vi "sub_breakdown-check.vi"(7 "breakdown type":T1=enum."input pwr", 8 "error in (no error)":errorcluster) -> (0 "error out":errorcluster)   [LabVIEW 2019]
uses:
  breakdown.ctl
  _ctrl/rw.ctl
  _ctrl/init-r-w.ctl
  SubVIs/common/_ctrl/system-status.ctl
  _ctrl/DSP_action.ctl
  _ctrl/create-rw-close.ctl
  _ctrl/start.ctl
  common/shutdown-type.ctl
  Devices/NI Board/cDAQ-9476 DO/cnt_Relay.ctl
  SubVIs/common/hw-control.ctl
  SubVIs/common/cmd_tablecnt.ctl
  SubVIs/count/cmd_count.ctl
  SubVIs/common/Glob_Ref.vi
  common/Global_params.vi
panel:
  out "부하전압":dbl
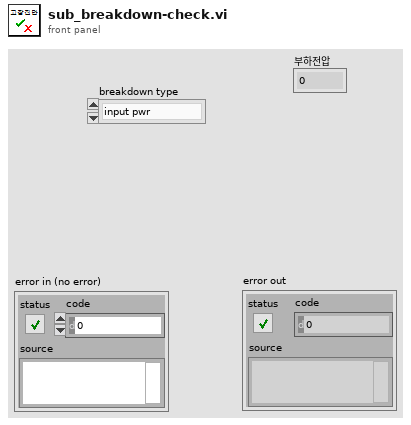
[diagram p1: front panel]
types:
  T1 = typedef "breakdown.ctl" = enum16{"DL950 items", "input pwr", "output pwr", "output pwr_adv"}
  T2 = typedef "rw.ctl" = enum16{"read", "write"}
  T3 = typedef "Breakdown-Spec.ctl" = cluster{"제어단 단선 Irms[mA](이하)":dbl, "제어단 특성 전류 Irms[mA] Max":dbl, "제어단 특성 전류 Irms[mA] Min":dbl, "출력단 단선 Irms[mA](이하)":dbl, "출력단 특성 전류 Irms[mA]  Max":dbl, "출력단 특성전류 Irms[mA]  Min":dbl, "온도[degree]":dbl}
  T4 = typedef "Testing-info.ctl" = cluster{"전체채널수":u8, "현재채널번호":u8, "Irms":dbl, "입력전압":dbl, "입력전류":dbl, "출력전압":dbl, "출력전류":dbl, "온도":dbl, "제어단 단선":bool, "제어단 단락":bool, "제어단 특성변화":bool, "출력단 단선":bool, "출력단 단락":bool, "출력단 특성변화":bool, "출력단 전압":bool, "카운트 일치":bool, "Irms 판정":bool, "온도":bool, "테스트 회수":u32, "TestType":T5, "현재회수":u32, "Ch selection":cluster{"1ch":bool, "2ch":bool, "3ch":bool, "4ch":bool, "5ch":bool, "6ch":bool}, "반복":u32, "Path":path, "파일생성주기":u32, "start time":dbl, "stop time":dbl, "현재반복회수":u32, "NG":cluster{"입출력 카운트":bool, "출력전류RMS":bool}}
  T5 = typedef "sequence_single.ctl" = enum16{"Register", "RC", "B1", "B2", "B3", "Oper_LV", "Oper_HV", "ContR_LV"}
  T6 = typedef "init-r-w.ctl" = enum16{"init", "read", "write"}
  T7 = typedef "DSP_action.ctl" = enum16{"False", "cont", "on", "off", "discont", "protection", "protection_seq", "preread", "level_seq", "level_m", "read", "stop", "exit"}
  T8 = typedef "start.ctl" = enum16{"init", "open", "set", "start", "stop", "read", "read_items", "query", "close", "T_single", "reset", "exit"}
  T9 = typedef "create-rw-close.ctl" = enum16{"create", "write", "read", "delete", "close"}
  T10 = typedef "shutdown-type.ctl" = enum16{"soft", "all"}
  T11 = typedef "system-status.ctl" = enum16{"Initial", "Update", "Clear", "Read"}
  T12 = typedef "cnt_Relay.ctl" = enum32{"R_Load", "R_out1", "R_out2", "R_out3", "R_out4", "R_out5", "R_out6", "R8", "R9", "R10", "R11", "R12", "R13", "R14", "R15", "R16", "R_in1", "R_in2", "R_in3", "R_in4", "R_in5", "R_in6", "R23", "R24", "R25", "R26", "R27", "R_red", "R_yellow", "R_green", "R_buz", "R_purple"}
  T13 = typedef "cmd_count.ctl" = enum16{"init", "count", "default"}
  T14 = typedef "cmd_tablecnt.ctl" = enum16{"Create", "Inital", "Write", "Default"}
  T15 = typedef "DSP_retrun.ctl" = cluster{"voltage":dbl, "current":dbl, "Read Data":string}
  T16 = typedef "error_rc.ctl" = cluster{"제어단 단선":bool, "제어단 단락":bool, "제어단 특성변화":bool, "출력단 단선":bool, "출력단 단락":bool, "출력단 특성변화":bool, "출력전압":bool, "카운트 일치":bool, "전압 98%":bool, "전압 63%":bool, "전류 37%":bool, "방전전압":bool, "온도":bool}
  T17 = typedef "cap_config.ctl" = cluster{"Test Mode":T18, "ON time[ms]":dbl, "OFF time[ms]":dbl, "1. 작동시간[분]":dbl, "2. 미작동시간[분]":dbl, "3. 작동시간[분]":dbl, "level[V]":dbl, "duty":dbl, "Freq":dbl, "Voltage+[V]":dbl, "Voltage-[V]":dbl, "Current+[A]":dbl, "Current-[A]":dbl, "출력전압[V]":dbl, "출력전류[A]":dbl, "OVP Level":dbl, "OCP Level":dbl, "Time Div":u16, "Record Len":i32, "방전 기준[V]":dbl, "Repeate (Each Ch)":u32, "Cycle[N]":u32, "작동간격[분]":dbl, "TrigPos[%]":dbl, "시험시간[분]":dbl}
  T18 = typedef "시험모드선택.ctl" = enum16{"6.3.1 온도방치 시험", "6.3.2 저온 작동/방치 시험", "6.3.3 고온 작동/방치 시험", "6.3.4 온도 싸이클 시험", "6.3.6 온습도 싸이클 시험", "6.3.7 고온고습 방치", "6.3.8 결로 시험", "6.3.9 빙결시험", "6.3.10 공진", "6.3.11.1 작동가진", "6.3.11.2 비작동 가진 ", "6.3.12 충격시험"}
  T19 = typedef "hw-control.ctl" = enum16{"DL950 ready", "DL950 clear", "DL950 trigger", "DL950 read", "DL950 read seq", "DL950 Tsingle query", "AO 12v", "AO wave", "AO 0v", "relay all-off", "Discharge check", "Discharge", "Relay1", "Relay2", "Relay3", "Relay4", "Relay5", "Relay6", "BP4610 onoff", "BP4610 set", "DSP1500 set", "DSP1500 onoff"}
  T20 = typedef "Judge_RC.ctl" = cluster{"전압 63%[mS] Min":dbl, "전압 98%[mS] Min":dbl, "전류 37%[mS] Min":dbl, "접촉저항[mOhm] Min":dbl, "출력전류 Irms[mA] Min":dbl, "전압 63%[mS] Max":dbl, "전압 98%[mS] Max":dbl, "전류 37%[mS] Max":dbl, "접촉저항[mOhm] Max":dbl, "출력전류 Irms[mA] Max":dbl}
  T21 = typedef "measure_reg.ctl" = cluster{"입력카운트":dbl, "출력카운트":dbl, "부하전압 RMS":dbl, "입력전류 RMS":dbl, "출력전류 RMS":dbl, "온도":dbl, "부하전압(고장)":dbl}
  T22 = typedef "measure_rc.ctl" = cluster{"입력카운트":dbl, "출력카운트":dbl, "Rising Time 63%":dbl, "Rising Time 98%":dbl, "Failing Time 37%":dbl, "입력전류 RMS":dbl, "출력전류 RMS":dbl, "출력전압 + 평균 63%":dbl, "출력전압 - 평균 63%":dbl, "출력전류 평균 63%":dbl, "접촉저항":dbl, "온도":dbl, "방전전압":dbl, "부하전압(고장)":dbl, "충전전압 63초":dbl, "충전전압 98초":dbl, "충전전류 37초":dbl, "전압강하":dbl}
  T23 = typedef "data_contR.ctl" = cluster{"입력카운트":dbl, "출력카운트":dbl, "입력전류 RMS":dbl, "출력전류 RMS":dbl, "출력전압(+)_Avg":dbl, "출력전압(-)_Avg":dbl, "출력전류_Avg":dbl, "접촉저항":dbl, "온도":dbl, "부하전압":dbl}
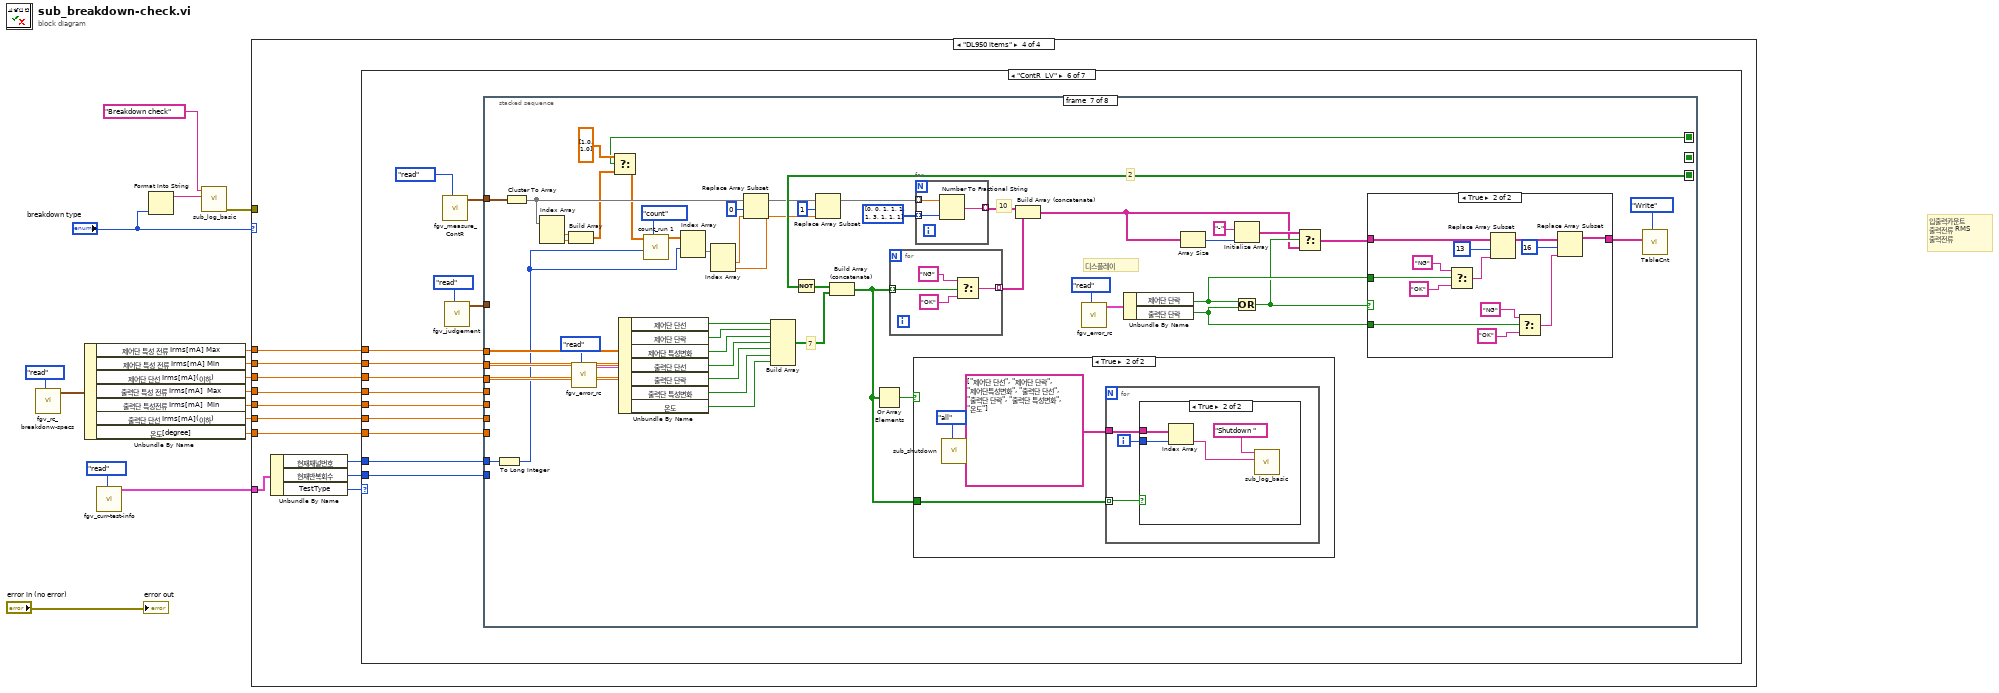
[diagram p0: block diagram]
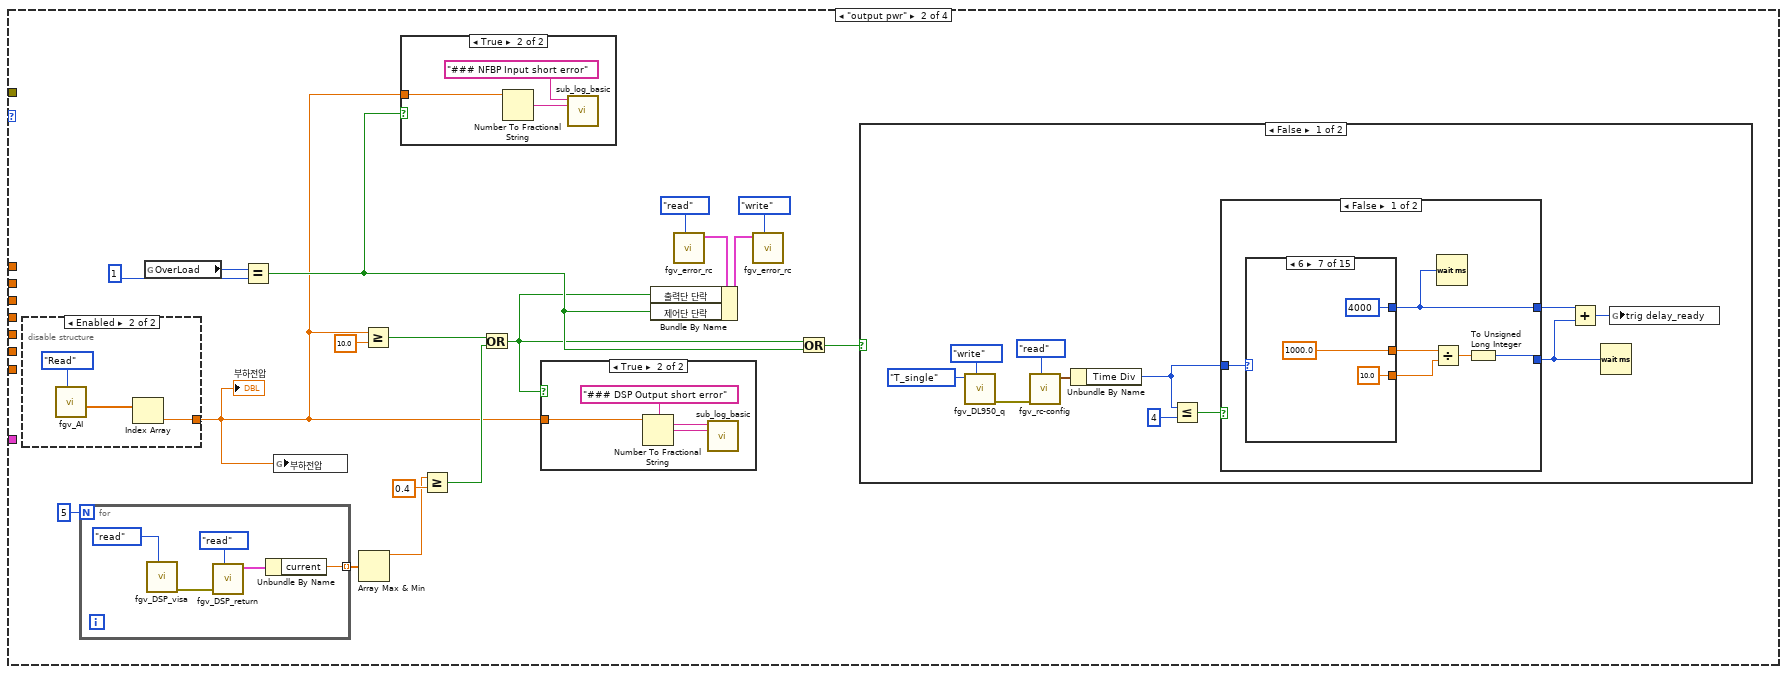
[diagram p3: hidden frame]
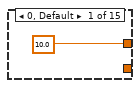
[diagram p4: hidden frame]
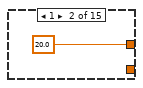
[diagram p5: hidden frame]
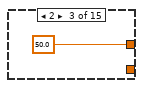
[diagram p6: hidden frame]
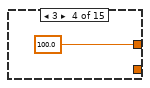
[diagram p7: hidden frame]
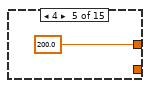
[diagram p8: hidden frame]
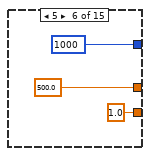
[diagram p9: hidden frame]
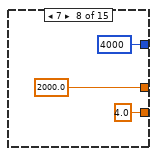
[diagram p10: hidden frame]
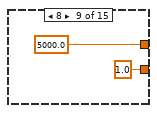
[diagram p11: hidden frame]
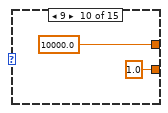
[diagram p12: hidden frame]
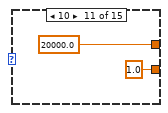
[diagram p13: hidden frame]
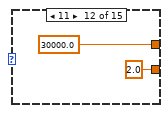
[diagram p14: hidden frame]
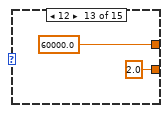
[diagram p15: hidden frame]
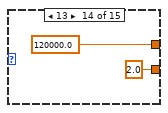
[diagram p16: hidden frame]
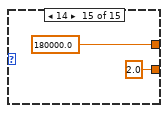
[diagram p17: hidden frame]
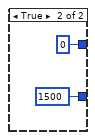
[diagram p18: hidden frame]
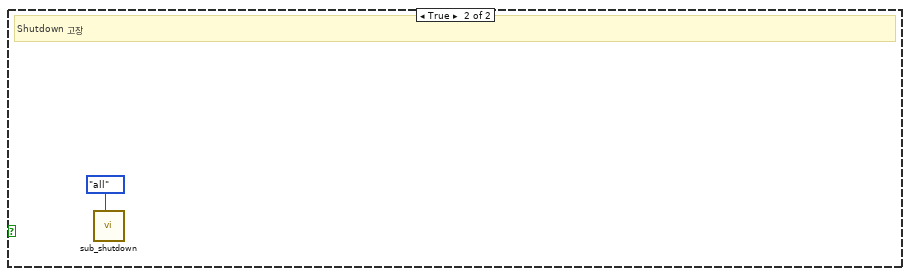
[diagram p19: hidden frame]
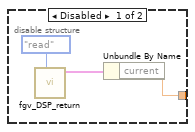
[diagram p20: hidden frame]
diagram:
  # "입출력카운트\n출력전류 RMS\n출력전류"
  n1 = call "fgv_rc_breakdonw-specs.vi"("cmd"=rw."read") -> ("BreakdownSpec 2"=w7:T3)  [unwired: 10 in]
  n2 = Unbundle By Name(w7) -> ("제어단 특성 전류 Irms[mA] Max"=w10:dbl, "제어단 특성 전류 Irms[mA] Min"=w9:dbl, "제어단 단선 Irms[mA](이하)"=w8:dbl, "출력단 특성 전류 Irms[mA]  Max"=w5:dbl, "출력단 특성전류 Irms[mA]  Min"=w4:dbl, "출력단 단선 Irms[mA](이하)"=w3:dbl, "온도[degree]"=w2:dbl)
  n3 = call "fgv_curr-test-info.vi"("cmd"=rw."read") -> ("현재테스트 정보 2"=w6:T4)  [unwired: 10 in]
  n4 = Format Into String("breakdown type") -> (resulting string=w13:string)  [unwired: 3 in, 1 out]
  n5 = call "sub_log_basic.vi"("desc"=w13, "Title"="Breakdown check") -> ("error out"=w12:errorcluster)  [unwired: 9 in]
  n6 = case shown="\"DL950 items\"" "breakdown type" {
    tunnel: w12 -> [_ _ _ _]
    tunnel: w10 -> [_ _ _ w214]
    tunnel: w9 -> [_ _ _ w213]
    tunnel: w8 -> [_ _ _ w212]
    tunnel: w6 -> [_ _ w123 w211]
    tunnel: w5 -> [_ _ _ w209]
    tunnel: w4 -> [_ _ _ w208]
    tunnel: w3 -> [_ _ _ w207]
    tunnel: w2 -> [_ _ _ w206]
    frame "input pwr", Default {
    }
    frame "output pwr" {
      n7 = disable-structure shown="Enabled" {
        disable-tunnel: [w87 w90] -> w17
        frame Disabled {
          n8 = call "fgv_DSP_return.vi"("cmd"=rw."read") -> ("return 2"=w88:T15)  [unwired: 9 in, 1 out]
          n9 = Unbundle By Name(w88) -> ("current"=w87:dbl)
        }
        frame Enabled {
          n10 = call "fgv_AI.vi"("Mode"=system-status."Read") -> ("mean-vals"=w92:dbl[])  [unwired: 8 in, 2 out]
          n11 = Index Array(array=w92) -> (element=w90:dbl)  [unwired: 1 in]
        }
      }
      "부하전압" <- w17
      n12 = for {
        N: 5 -> [_]
        tunnel: [w34] -> w23 mode=indexing
        n13 = call "fgv_DSP_visa.vi"("action"=DSP_action."read") -> ("error out"=w35:errorcluster)  [unwired: 10 in]
        n14 = call "fgv_DSP_return.vi"("cmd"=rw."read", "error in (no error)"=w35) -> ("return 2"=w36:T15)  [unwired: 8 in, 1 out]
        n15 = Unbundle By Name(w36) -> ("current"=w34:dbl)
      }
      n16 = global read "Glob_Ref.vi" "OverLoad"() -> (w28:i32)
      n17 = Equal?(x=w28, y=1) -> (x = y?=w26:bool)
      n18 = global write "Glob_Ref.vi" "부하전압"(w17) -> ()
      n19 = Array Max & Min(array=w23) -> (max value=w21:dbl)  [unwired: 3 out]
      n20 = Greater Or Equal?(x=w17, y=10.0) -> (x >= y?=w20:bool)
      n21 = case shown="True" w26 {
        tunnel: w17 -> [_ w96]
        frame False {
        }
        frame True {
          n22 = Number To Fractional String(number=w96) -> (F-format string=w97:string)  [unwired: 3 in]
          n23 = call "sub_log_basic.vi"("desc"=w97, "Title"="### NFBP Input short error") -> ()  [unwired: 9 in, 1 out]
        }
      }
      n24 = Greater Or Equal?(x=w21, y=0.4) -> (x >= y?=w19:bool)
      n25 = Or(x=w20, y=w19) -> (x .or. y?=w18:bool)
      n26 = case shown="True" w18 {
        tunnel: w17 -> [_ w93]
        frame False {
        }
        frame True {
          n27 = Number To Fractional String(number=w93) -> (F-format string=w94:string)  [unwired: 3 in]
          n28 = call "sub_log_basic.vi"("desc"=w94, "Title"="### DSP Output short error") -> ()  [unwired: 9 in, 1 out]
        }
      }
      n29 = call "fgv_error_rc.vi"("cmd"=init-r-w."read") -> ("Error 2"=w33:T16)  [unwired: 10 in]
      n30 = Bundle By Name(cluster=w33, "출력단 단락"=w18, "제어단 단락"=w26) -> (w32:T16)
      n31 = call "fgv_error_rc.vi"("cmd"=init-r-w."write", "Error"=w32) -> ()  [unwired: 9 in, 1 out]
      n32 = Or(x=w18, y=w26) -> (x .or. y?=w25:bool)
      n33 = case shown="False" w25 {
        frame False {
          n34 = call "fgv_DL950_q.vi"("cmd"=create-rw-close."write", "data"=start."T_single") -> ("error out"=w45:errorcluster)  [unwired: 8 in, 1 out]
          n35 = call "fgv_rc-config.vi"("cmd"=rw."read", "error in (no error)"=w45) -> ("Testconfig out"=w47:T17)  [unwired: 8 in, 1 out]
          n36 = Unbundle By Name(w47) -> ("Time Div"=w42:u16)
          n37 = Less Or Equal?(x=w42, y=u16 4) -> (x <= y?=w43:bool)
          n38 = case shown="False" w43 {
            tunnel: [w55 u32 1500] -> w40
            tunnel: w42 -> [w54 _]
            tunnel: [w50 u32 0 ("milliseconds to wait")] -> w41
            frame False {
              n39 = case shown="6" w54 {
                tunnel: [10.0 ("number") 20.0 ("number") 50.0 ("number") 100.0 ("number") 200.0 ("number") 500.0 ("number") 1000.0 ("number") 2000.0 ("number") 5000.0 ("number") 10000.0 ("number") 20000.0 ("number") 30000.0 ("number") 60000.0 ("number") 120000.0 ("number") 180000.0 ("number")] -> w53
                tunnel: [_ _ _ _ _ u32 1000 ("milliseconds to wait") u32 4000 ("milliseconds to wait") u32 4000 ("milliseconds to wait") _ _ _ _ _ _ _] -> w50
                tunnel: [_ _ _ _ _ 1.0 ("y") 10.0 ("y") 4.0 ("y") 1.0 ("y") 1.0 ("y") 1.0 ("y") 2.0 ("y") 2.0 ("y") 2.0 ("y") 2.0 ("y")] -> w51
                frame 0, Default {
                }
                frame 1 {
                }
                frame 2 {
                }
                frame 3 {
                }
                frame 4 {
                }
                frame 5 {
                }
                frame 6 {
                }
                frame 7 {
                }
                frame 8 {
                }
                frame 9 {
                }
                frame 10 {
                }
                frame 11 {
                }
                frame 12 {
                }
                frame 13 {
                }
                frame 14 {
                }
              }
              n40 = Divide(x=w53, y=w51) -> (x/y=w52:dbl)
              n41 = Wait (ms)(milliseconds to wait=w50) -> ()  [unwired: 1 out]
              n42 = To Unsigned Long Integer(number=w52) -> (unsigned 32bit integer=w55:u32)
            }
            frame True {
            }
          }
          n43 = Add(x=w41, y=w40) -> (x+y=w39:u32)
          n44 = Wait (ms)(milliseconds to wait=w40) -> ()  [unwired: 1 out]
          n45 = global write "Global_params.vi" "trig delay_ready"(w39) -> ()
        }
        frame True {
          # "Shutdown 고장"
          n46 = call "sub_shutdown.vi"("type"=shutdown-type."all") -> ()  [unwired: 10 in, 1 out]
        }
      }
    }
    frame "output pwr_adv" {
      n47 = disable-structure shown="Enabled" {
        disable-tunnel: [w198 w201] -> w106
        frame Disabled {
          n48 = call "fgv_DSP_return.vi"("cmd"=rw."read") -> ("return 2"=w199:T15)  [unwired: 9 in, 1 out]
          n49 = Unbundle By Name(w199) -> ("current"=w198:dbl)
        }
        frame Enabled {
          n50 = call "fgv_AI.vi"("Mode"=system-status."Read") -> ("mean-vals"=w203:dbl[])  [unwired: 8 in, 2 out]
          n51 = Index Array(array=w203) -> (element=w201:dbl)  [unwired: 1 in]
        }
      }
      n52 = for {
        N: 5 -> [_]
        tunnel: [w125] -> w112 mode=indexing
        tunnel: [w124] -> w100
        n53 = call "fgv_DSP_visa.vi"("action"=DSP_action."read") -> ("error out"=w126:errorcluster)  [unwired: 10 in]
        n54 = call "fgv_DSP_return.vi"("cmd"=rw."read", "error in (no error)"=w126) -> ("error out"=w124:errorcluster, "return 2"=w127:T15)  [unwired: 8 in]
        n55 = Unbundle By Name(w127) -> ("current"=w125:dbl)
      }
      n56 = global read "Glob_Ref.vi" "OverLoad"() -> (w117:i32)
      n57 = Equal?(x=w117, y=1) -> (x = y?=w115:bool)
      n58 = Unbundle By Name(w123) -> ("현재채널번호"=w103:u8)
      n59 = global write "Glob_Ref.vi" "부하전압"(w106) -> ()
      n60 = Array Max & Min(array=w112) -> (max value=w110:dbl)  [unwired: 3 out]
      n61 = Greater Or Equal?(x=w106, y=10.0) -> (x >= y?=w109:bool)
      n62 = case shown="True" w115 {
        tunnel: w106 -> [_ w192]
        frame False {
        }
        frame True {
          n63 = Number To Fractional String(number=w192) -> (F-format string=w193:string)  [unwired: 3 in]
          n64 = call "sub_log_basic.vi"("desc"=w193, "Title"="### NFBP Input short error") -> ()  [unwired: 9 in, 1 out]
        }
      }
      n65 = case shown="0, Default" w103 {
        tunnel: [cnt_Relay."R_out1" ("Relay") cnt_Relay."R_out2" ("Relay") cnt_Relay."R_out3" ("Relay") _ _ _] -> w102
        frame 0, Default {
        }
        frame 1 {
        }
        frame 2 {
        }
        frame 3 {
          (unwired) hw-control."Relay4" ("cmd")
        }
        frame 4 {
          (unwired) hw-control."Relay5" ("cmd")
        }
        frame 5 {
          (unwired) hw-control."Relay6" ("cmd")
        }
      }
      n66 = Greater Or Equal?(x=w110, y=0.4) -> (x >= y?=w108:bool)
      n67 = Or(x=w109, y=w108) -> (x .or. y?=w107:bool)
      n68 = case shown="True" w107 {
        tunnel: w106 -> [_ w189]
        frame False {
        }
        frame True {
          n69 = Number To Fractional String(number=w189) -> (F-format string=w190:string)  [unwired: 3 in]
          n70 = call "sub_log_basic.vi"("desc"=w190, "Title"="### DSP Output short error") -> ()  [unwired: 9 in, 1 out]
        }
      }
      n71 = call "fgv_DSP_visa.vi"("action"=DSP_action."off", "error in"=w100) -> ("error out"=w99:errorcluster)  [unwired: 9 in]
      n72 = call "fgv_error_rc.vi"("cmd"=init-r-w."read") -> ("Error 2"=w122:T16)  [unwired: 10 in]
      n73 = Bundle By Name(cluster=w122, "출력단 단락"=w107, "제어단 단락"=w115) -> (w121:T16)
      n74 = call "fgv_error_rc.vi"("cmd"=init-r-w."write", "Error"=w121) -> ()  [unwired: 9 in, 1 out]
      n75 = Or(x=w107, y=w115) -> (x .or. y?=w114:bool)
      n76 = call "sub ch-val-global.vi"("Relay"=w102, "error in (no error)"=w99, "onoff"=FALSE) -> ("error out"=w104:errorcluster)  [unwired: 8 in]
      n77 = case shown="False" w114 {
        tunnel: w104 -> [w137 _]
        tunnel: w102 -> [w132 _]
        frame False {
          n78 = call "fgv_DL950_q.vi"("cmd"=create-rw-close."write", "error in"=w137, "data"=start."T_single") -> ("error out"=w144:errorcluster)  [unwired: 7 in, 1 out]
          n79 = call "fgv_rc-config.vi"("cmd"=rw."read", "error in (no error)"=w144) -> ("error out"=w134:errorcluster, "Testconfig out"=w146:T17)  [unwired: 8 in]
          n80 = Unbundle By Name(w146) -> ("Time Div"=w141:u16)
          n81 = Less Or Equal?(x=w141, y=u16 4) -> (x <= y?=w142:bool)
          n82 = case shown="False" w142 {
            tunnel: [w157 u32 1500] -> w139
            tunnel: w141 -> [w156 _]
            tunnel: [w152 u32 0 ("milliseconds to wait")] -> w140
            frame False {
              n83 = case shown="6" w156 {
                tunnel: [10.0 ("number") 20.0 ("number") 50.0 ("number") 100.0 ("number") 200.0 ("number") 500.0 ("number") 1000.0 ("number") 2000.0 ("number") 5000.0 ("number") 10000.0 ("number") 20000.0 ("number") 30000.0 ("number") 60000.0 ("number") 120000.0 ("number") 180000.0 ("number")] -> w155
                tunnel: [_ _ _ _ _ u32 1000 ("milliseconds to wait") u32 4000 ("milliseconds to wait") u32 4000 ("milliseconds to wait") _ _ _ _ _ _ _] -> w152
                tunnel: [_ _ _ _ _ 1.0 ("y") 10.0 ("y") 4.0 ("y") 1.0 ("y") 1.0 ("y") 1.0 ("y") 2.0 ("y") 2.0 ("y") 2.0 ("y") 2.0 ("y")] -> w153
                frame 0, Default {
                }
                frame 1 {
                }
                frame 2 {
                }
                frame 3 {
                }
                frame 4 {
                }
                frame 5 {
                }
                frame 6 {
                }
                frame 7 {
                }
                frame 8 {
                }
                frame 9 {
                }
                frame 10 {
                }
                frame 11 {
                }
                frame 12 {
                }
                frame 13 {
                }
                frame 14 {
                }
              }
              n84 = Divide(x=w155, y=w153) -> (x/y=w154:dbl)
              n85 = Wait (ms)(milliseconds to wait=w152) -> ()  [unwired: 1 out]
              n86 = To Unsigned Long Integer(number=w154) -> (unsigned 32bit integer=w157:u32)
            }
            frame True {
            }
          }
          n87 = Add(x=w140, y=w139) -> (x+y=w138:u32)
          n88 = flat-sequence {
            tunnel: w139 -> [w151]
            tunnel: [w150] -> w135
            tunnel: w134 -> [w150]
            tunnel: [w149] -> w133
            tunnel: w132 -> [w149]
            frame #0 {
              n89 = Wait (ms)(milliseconds to wait=w151) -> ()  [unwired: 1 out]
            }
          }
          n90 = global write "Global_params.vi" "trig delay_ready"(w138) -> ()
          n91 = call "sub ch-val-global.vi"("Relay"=w133, "error in (no error)"=w135, "onoff"=TRUE) -> ("error out"=w130:errorcluster)  [unwired: 8 in]
          n92 = call "fgv_DSP_visa.vi"("action"=DSP_action."on", "error in"=w130) -> ()  [unwired: 9 in, 1 out]
        }
        frame True {
          # "Shutdown 고장"
          n93 = call "sub_shutdown.vi"("type"=shutdown-type."all") -> ()  [unwired: 10 in, 1 out]
        }
      }
    }
    frame "DL950 items" {
      n94 = Unbundle By Name(w211) -> ("현재채널번호"=w204:u8, "현재반복회수"=w205:u32, "TestType"=w210:T5)
      n95 = case shown="\"ContR_LV\"" w210 {
        tunnel: w214 -> [w227 w439 w675 w887 w1099 w1317 w1536]
        tunnel: w213 -> [w226 w438 w674 w886 w1098 w1316 w1535]
        tunnel: w212 -> [w225 w437 w673 w885 w1097 w1315 w1534]
        tunnel: w209 -> [w224 w436 w672 w884 w1096 w1314 w1533]
        tunnel: w208 -> [w223 w435 w671 w883 w1095 w1313 w1532]
        tunnel: w207 -> [w222 w434 w670 w882 w1094 w1312 w1531]
        tunnel: w206 -> [w221 w433 w669 w881 w1093 w1311 w1530]
        tunnel: w205 -> [w220 w432 w668 w880 w1092 w1310 w1529]
        tunnel: w204 -> [w217 w429 w665 w877 w1089 w1307 w1526]
        frame "Register", Default {
          n96 = call "fgv_judgement.vi"("cmd"=rw."read") -> ("Test Judgement 2"=w218:T20)  [unwired: 9 in, 1 out]
          n97 = call "fgv_measure_reg.vi"("cmd"=rw."read") -> ("measure_reg 2"=w215:T21)  [unwired: 10 in]
          n98 = stacked-sequence {
            seq-local: [_ _ _ _ _ w338 _ _] -> [_ _ _ _ _ _ w392 _]
            tunnel: w227 -> [w240 _ _ _ _ _ _ _]
            tunnel: w226 -> [w239 _ _ _ _ _ _ _]
            tunnel: w225 -> [_ w258 _ _ _ _ _ _]
            tunnel: w224 -> [_ _ w273 _ _ _ _ _]
            tunnel: w223 -> [_ _ w272 _ _ _ _ _]
            tunnel: w222 -> [_ _ _ w292 _ _ _ _]
            tunnel: w221 -> [_ _ _ _ w311 _ _ _]
            tunnel: w220 -> [_ _ _ _ _ w347 _ _]
            tunnel: w218 -> [_ _ _ _ _ w346 _ _]
            tunnel: w217 -> [_ _ _ _ _ _ w352 w424]
            tunnel: w215 -> [w233 w253 w271 w291 w310 w345 w388 _]
            frame #0 {
              n99 = Unbundle By Name(w233) -> ("입력전류 RMS"=w230:dbl)
              n100 = In Range and Coerce(upper limit=w240, x=w230, lower limit=w239) -> (In Range?=w238:bool)  [unwired: 1 out]
              n101 = Not(x=w238) -> (.not. x?=w229:bool)
              n102 = Not A Number/Path/Refnum?(number/path/refnum=w230) -> (NaN/Path/Refnum?=w232:bool)
              n103 = Select(t=TRUE, s=w232, f=w229) -> (s? t:f=w228:bool)
              n104 = case shown="True" w228 {
                tunnel: w230 -> [_ w245]
                frame False {
                }
                frame True {
                  n105 = Number To Fractional String(number=w245) -> (F-format string=w246:string)  [unwired: 3 in]
                  n106 = call "sub_log_basic.vi"("desc"=w246, "Title"="### DL950 input curr spec out ") -> ()  [unwired: 9 in, 1 out]
                }
              }
              n107 = case shown="True" w228 {
                tunnel: w230 -> [_ w241]
                frame False {
                }
                frame True {
                  n108 = Number To Fractional String(number=w241) -> (F-format string=w242:string)  [unwired: 3 in]
                  n109 = call "fgv_status-display.vi"("Mode"=system-status."Update", "detail"=w242, "title"="Input RMS") -> ()  [unwired: 8 in, 1 out]
                }
              }
              n110 = call "fgv_error_rc.vi"("cmd"=init-r-w."read") -> ("Error 2"=w237:T16)  [unwired: 10 in]
              n111 = Bundle By Name(cluster=w237, "제어단 특성변화"=w228) -> (w236:T16)
              n112 = call "fgv_error_rc.vi"("cmd"=init-r-w."write", "Error"=w236) -> ()  [unwired: 9 in, 1 out]
            }
            frame #1 {
              n113 = Unbundle By Name(w253) -> ("입력전류 RMS"=w250:dbl)
              n114 = Less Or Equal?(x=w250, y=w258) -> (x <= y?=w249:bool)
              n115 = Not A Number/Path/Refnum?(number/path/refnum=w250) -> (NaN/Path/Refnum?=w252:bool)
              n116 = Select(t=TRUE, s=w252, f=w249) -> (s? t:f=w248:bool)
              n117 = call "fgv_error_rc.vi"("cmd"=init-r-w."read") -> ("Error 2"=w256:T16)  [unwired: 10 in]
              n118 = Bundle By Name(cluster=w256, "제어단 단선"=w248) -> (w257:T16)
              n119 = case shown="True" w248 {
                tunnel: w258 -> [_ w263]
                frame False {
                }
                frame True {
                  n120 = Number To Fractional String(number=w263) -> (F-format string=w264:string)  [unwired: 3 in]
                  n121 = call "sub_log_basic.vi"("desc"=w264, "Title"="### DL950 input open") -> ()  [unwired: 9 in, 1 out]
                }
              }
              n122 = case shown="True" w248 {
                tunnel: w250 -> [_ w259]
                frame False {
                }
                frame True {
                  n123 = Number To Fractional String(number=w259) -> (F-format string=w260:string)  [unwired: 3 in]
                  n124 = call "fgv_status-display.vi"("Mode"=system-status."Update", "detail"=w260, "title"="Input RMS") -> ()  [unwired: 8 in, 1 out]
                }
              }
              n125 = call "fgv_error_rc.vi"("cmd"=init-r-w."write", "Error"=w257) -> ()  [unwired: 9 in, 1 out]
            }
            frame #2 {
              n126 = Unbundle By Name(w271) -> ("출력전류 RMS"=w268:dbl)
              n127 = In Range and Coerce(upper limit=w273, x=w268, lower limit=w272) -> (In Range?=w278:bool)  [unwired: 1 out]
              n128 = Not(x=w278) -> (.not. x?=w267:bool)
              n129 = Not A Number/Path/Refnum?(number/path/refnum=w268) -> (NaN/Path/Refnum?=w270:bool)
              n130 = Select(t=TRUE, s=w270, f=w267) -> (s? t:f=w266:bool)
              n131 = case shown="True" w266 {
                tunnel: w268 -> [_ w283]
                frame False {
                }
                frame True {
                  n132 = Number To Fractional String(number=w283) -> (F-format string=w284:string)  [unwired: 3 in]
                  n133 = call "sub_log_basic.vi"("desc"=w284, "Title"="### DL950 output curr spec out ") -> ()  [unwired: 9 in, 1 out]
                }
              }
              n134 = case shown="True" w266 {
                tunnel: w268 -> [_ w279]
                frame False {
                }
                frame True {
                  n135 = Number To Fractional String(number=w279) -> (F-format string=w280:string)  [unwired: 3 in]
                  n136 = call "fgv_status-display.vi"("Mode"=system-status."Update", "detail"=w280, "title"="Output RMS") -> ()  [unwired: 8 in, 1 out]
                }
              }
              n137 = call "fgv_error_rc.vi"("cmd"=init-r-w."read") -> ("Error 2"=w277:T16)  [unwired: 10 in]
              n138 = Bundle By Name(cluster=w277, "출력단 특성변화"=w266) -> (w276:T16)
              n139 = call "fgv_error_rc.vi"("cmd"=init-r-w."write", "Error"=w276) -> ()  [unwired: 9 in, 1 out]
            }
            frame #3 {
              n140 = Unbundle By Name(w291) -> ("출력전류 RMS"=w287:dbl)
              n141 = Less Or Equal?(x=w287, y=w292) -> (x <= y?=w288:bool)
              n142 = Not A Number/Path/Refnum?(number/path/refnum=w287) -> (NaN/Path/Refnum?=w290:bool)
              n143 = Select(t=TRUE, s=w290, f=w288) -> (s? t:f=w286:bool)
              n144 = case shown="True" w286 {
                tunnel: w292 -> [_ w301]
                frame False {
                }
                frame True {
                  n145 = Number To Fractional String(number=w301) -> (F-format string=w302:string)  [unwired: 3 in]
                  n146 = call "sub_log_basic.vi"("desc"=w302, "Title"="### DL950 output open") -> ()  [unwired: 9 in, 1 out]
                }
              }
              n147 = case shown="True" w286 {
                tunnel: w287 -> [_ w297]
                frame False {
                }
                frame True {
                  n148 = Number To Fractional String(number=w297) -> (F-format string=w298:string)  [unwired: 3 in]
                  n149 = call "fgv_status-display.vi"("Mode"=system-status."Update", "detail"=w298, "title"="Output RMS") -> ()  [unwired: 8 in, 1 out]
                }
              }
              n150 = call "fgv_error_rc.vi"("cmd"=init-r-w."read") -> ("Error 2"=w295:T16)  [unwired: 10 in]
              n151 = Bundle By Name(cluster=w295, "출력단 단선"=w286) -> (w296:T16)
              n152 = call "fgv_error_rc.vi"("cmd"=init-r-w."write", "Error"=w296) -> ()  [unwired: 9 in, 1 out]
            }
            frame #4 {
              n153 = Unbundle By Name(w310) -> ("온도"=w307:dbl)
              n154 = Less Or Equal?(x=w307, y=w311) -> (x <= y?=w306:bool)
              n155 = Not(x=w306) -> (.not. x?=w305:bool)
              n156 = Not A Number/Path/Refnum?(number/path/refnum=w307) -> (NaN/Path/Refnum?=w309:bool)
              n157 = Select(t=TRUE, s=w309, f=w305) -> (s? t:f=w304:bool)
              n158 = case shown="True" w304 {
                tunnel: w311 -> [_ w320]
                frame False {
                }
                frame True {
                  n159 = Number To Fractional String(number=w320) -> (F-format string=w321:string)  [unwired: 3 in]
                  n160 = call "sub_log_basic.vi"("desc"=w321, "Title"="### DL950 output open") -> ()  [unwired: 9 in, 1 out]
                }
              }
              n161 = case shown="True" w304 {
                tunnel: w307 -> [_ w316]
                frame False {
                }
                frame True {
                  n162 = Number To Fractional String(number=w316) -> (F-format string=w317:string)  [unwired: 3 in]
                  n163 = call "fgv_status-display.vi"("Mode"=system-status."Update", "detail"=w317, "title"="온도") -> ()  [unwired: 8 in, 1 out]
                }
              }
              n164 = call "fgv_error_rc.vi"("cmd"=init-r-w."read") -> ("Error 2"=w314:T16)  [unwired: 10 in]
              n165 = Bundle By Name(cluster=w314, "온도"=w304) -> (w315:T16)
              n166 = call "fgv_error_rc.vi"("cmd"=init-r-w."write", "Error"=w315) -> ()  [unwired: 9 in, 1 out]
            }
            frame #5 {
              n167 = Unbundle By Name(w346) -> ("출력전류 Irms[mA] Max"=w324:dbl, "출력전류 Irms[mA] Min"=w323:dbl)
              n168 = Unbundle By Name(w345) -> ("입력카운트"=w334:dbl, "출력카운트"=w330:dbl, "출력전류 RMS"=w327:dbl)
              n169 = To Double Precision Float(number=w347) -> ()  [unwired: 1 out]
              n170 = Equal?(x=w334, y=w330) -> (x = y?=w344:bool)
              n171 = In Range and Coerce(upper limit=w324, x=w327, lower limit=w323) -> (In Range?=w343:bool)  [unwired: 1 out]
              n172 = Build Array(w344, w343) -> (w338:bool[])
              n173 = Number To Fractional String(number=w327) -> (F-format string=w326:string)  [unwired: 3 in]
              n174 = call "sub_log_basic.vi"("desc"=w326, "Title"="출력전류") -> ("error out"=w325:errorcluster)  [unwired: 9 in]
              n175 = Number To Decimal String(number=w334) -> (decimal integer string=w333:string)  [unwired: 1 in]
              n176 = call "sub_log_basic.vi"("error in"=w325, "desc"=w333, "Title"="입력 카운트") -> ("error out"=w329:errorcluster)  [unwired: 8 in]
              n177 = Number To Decimal String(number=w330) -> (decimal integer string=w332:string)  [unwired: 1 in]
              n178 = call "sub_log_basic.vi"("error in"=w329, "desc"=w332, "Title"="출력 카운트") -> ()  [unwired: 8 in, 1 out]
              n179 = Not(x=w338) -> (.not. x?=w336:bool[])
              n180 = Array To Cluster(array=w336) -> (cluster=w337:cluster{"[0]":bool, "[1]":bool})
              n181 = call "fgv_curr-test-info.vi"("cmd"=rw."read") -> ("현재테스트 정보 2"=w340:T4)  [unwired: 10 in]
              n182 = Bundle By Name(cluster=w340, "NG"=w337) -> (w339:T4)
              n183 = call "fgv_curr-test-info.vi"("cmd"=rw."write", "현재테스트 정보"=w339) -> ()  [unwired: 9 in, 1 out]
            }
            frame #6 {
              # "디스플레이"
              n184 = To Long Integer(number=w352) -> (32bit integer=w351:i32)
              n185 = Cluster To Array(cluster=w388) -> (array=w353:dbl[])
              n186 = Index Array(array=w353) -> (element #1=w360:dbl, element #2=w359:dbl)  [unwired: 2 in]
              n187 = call "fgv_error_rc.vi"("cmd"=init-r-w."read") -> ("Error 2"=w379:T16)  [unwired: 10 in]
              n188 = Build Array(w360, w359) -> (w363:dbl[])
              n189 = Unbundle By Name(w379) -> ("제어단 단선"=w387:bool, "제어단 단락"=w386:bool, "제어단 특성변화"=w385:bool, "출력단 단선"=w384:bool, "출력단 단락"=w383:bool, "출력단 특성변화"=w382:bool, "온도"=w381:bool)
              n190 = call "count_run 1.vi"("cmd"=cmd_count."count", "CH"=w351, "Array_Count"=w363) -> ("Array_data"=w362:dbl[][])  [unwired: 7 in, 1 out]
              n191 = Index Array(array=w362, index (row)=w351) -> (element=w361:dbl[])  [unwired: 1 in]
              n192 = Index Array(array=w361) -> (element #1=w357:dbl, element #2=w354:dbl)  [unwired: 2 in]
              n193 = Replace Array Subset(array=w353, new element=w357, index=0) -> (w355:dbl[])
              n194 = Build Array(w387, w386, w385, w384, w383, w382, w381) -> (w377:bool[])
              n195 = Not(x=w392) -> (.not. x?=w378:bool[])
              n196 = Replace Array Subset(array=w355, new element=w354, index=1) -> (w349:dbl[])
              n197 = Build Array (concatenate)(w378, w377) -> (w365:bool[])
              n198 = Or Array Elements(Boolean array=w365) -> (logical OR=w389:bool)
              n199 = for {
                tunnel: w365 -> [w423] mode=indexing
                tunnel: [w420] -> w391 mode=indexing
                n200 = Select(t="NG", s=w423, f="OK") -> (s? t:f=w420:string)
              }
              n201 = case shown="True" w389 {
                tunnel: w365 -> [_ w411]
                frame False {
                }
                frame True {
                  n202 = call "sub_shutdown.vi"("type"=shutdown-type."all") -> ()  [unwired: 10 in, 1 out]
                  n203 = for {
                    tunnel: w411 -> [w415] mode=indexing
                    tunnel: string[] ["제어단 단선", "제어단 단락", "제어단특성변화", "출력단 단선", "출력단 단락", "출력단 특성변화", "온도"] -> [w414]
                    i -> [w413]
                    n204 = case shown="True" w415 {
                      tunnel: w414 -> [_ w418]
                      tunnel: w413 -> [_ w417]
                      frame False {
                      }
                      frame True {
                        n205 = Index Array(array=w418, index=w417) -> (element=w416:string)
                        n206 = call "sub_log_basic.vi"("desc"=w416, "Title"="Shutdown ") -> ()  [unwired: 9 in, 1 out]
                      }
                    }
                  }
                }
              }
              n207 = for {
                tunnel: [w395] -> w348 mode=indexing
                tunnel: w349 -> [w394] mode=indexing
                tunnel: i16[] [0, 0, 1, 1, 1, 1, 1] -> [w393] mode=indexing
                n208 = Number To Fractional String(number=w394, precision (6)=w393) -> (F-format string=w395:string)  [unwired: 2 in]
              }
              n209 = Build Array (concatenate)(w348, w391) -> (w367:string[])
              n210 = call "fgv_error_rc.vi"("cmd"=init-r-w."read") -> ("Error 2"=w375:T16)  [unwired: 10 in]
              n211 = Unbundle By Name(w375) -> ("제어단 단락"=w372:bool, "출력단 단락"=w371:bool)
              n212 = Array Size(array=w367) -> (size(s)=w373:i32)
              n213 = Initialize Array("-", w373) -> (w369:string[])
              n214 = Or(x=w372, y=w371) -> (x .or. y?=w370:bool)
              n215 = Select(t=w369, s=w370, f=w367) -> (s? t:f=w368:string[])
              n216 = case shown="True" w370 {
                tunnel: [w396 w407] -> w366
                tunnel: w368 -> [w396 w409]
                tunnel: w372 -> [_ w405]
                tunnel: w371 -> [_ w397]
                frame False {
                }
                frame True {
                  n217 = Select(t="NG", s=w405, f="OK") -> (s? t:f=w402:string)
                  n218 = Replace Array Subset(array=w409, new element=w402, index=9) -> (w408:string[])
                  n219 = Select(t="NG", s=w397, f="OK") -> (s? t:f=w398:string)
                  n220 = Replace Array Subset(array=w408, new element=w398, index=12) -> (w407:string[])
                }
              }
              n221 = call "TableCnt.vi"("cnt"=cmd_tablecnt."Write", "appended array"=w366) -> ()  [unwired: 8 in, 2 out]
            }
            frame #7 {
              # "저장"
              n222 = call "TableCnt.vi"("cnt"=cmd_tablecnt."Default") -> ("Item Names"=w425:string[][])  [unwired: 9 in, 1 out]
              n223 = Index Array(array=w425, index (col)=w424) -> ()  [unwired: 1 in, 1 out]
            }
          }
        }
        frame "RC", "B1" {
          n224 = call "fgv_judgement.vi"("cmd"=rw."read") -> ("Test Judgement 2"=w430:T20)  [unwired: 9 in, 1 out]
          n225 = call "fgv_measure_rc.vi"("cmd"=rw."read") -> ("measure_rc 2"=w427:T22)  [unwired: 10 in]
          n226 = stacked-sequence {
            seq-local: [_ _ _ _ _ w566 _ _] -> [_ _ _ _ _ _ w593 _]
            tunnel: w439 -> [w452 _ _ _ _ _ _ _]
            tunnel: w438 -> [w451 _ _ _ _ _ _ _]
            tunnel: w437 -> [_ w470 _ _ _ _ _ _]
            tunnel: w436 -> [_ _ w485 _ _ _ _ _]
            tunnel: w435 -> [_ _ w484 _ _ _ _ _]
            tunnel: w434 -> [_ _ _ w504 _ _ _ _]
            tunnel: w433 -> [_ _ _ _ w523 _ _ _]
            tunnel: w432 -> [_ _ _ _ _ w551 w615 _]
            tunnel: w430 -> [_ _ _ _ _ w567 _ _]
            tunnel: w429 -> [_ _ _ _ _ _ w585 _]
            tunnel: w427 -> [w445 w465 w483 w503 w522 w568 w594 _]
            frame #0 {
              n227 = Unbundle By Name(w445) -> ("입력전류 RMS"=w444:dbl)
              n228 = In Range and Coerce(upper limit=w452, x=w444, lower limit=w451) -> (In Range?=w450:bool)  [unwired: 1 out]
              n229 = Not(x=w450) -> (.not. x?=w442:bool)
              n230 = Not A Number/Path/Refnum?(number/path/refnum=w444) -> (NaN/Path/Refnum?=w443:bool)
              n231 = Select(t=TRUE, s=w443, f=w442) -> (s? t:f=w441:bool)
              n232 = case shown="True" w441 {
                tunnel: w444 -> [_ w457]
                frame False {
                }
                frame True {
                  n233 = Number To Fractional String(number=w457) -> (F-format string=w458:string)  [unwired: 3 in]
                  n234 = call "sub_log_basic.vi"("desc"=w458, "Title"="### DL950 input curr spec out ") -> ()  [unwired: 9 in, 1 out]
                }
              }
              n235 = case shown="True" w441 {
                tunnel: w444 -> [_ w453]
                frame False {
                }
                frame True {
                  n236 = Number To Fractional String(number=w453) -> (F-format string=w454:string)  [unwired: 3 in]
                  n237 = call "fgv_status-display.vi"("Mode"=system-status."Update", "detail"=w454, "title"="Input RMS") -> ()  [unwired: 8 in, 1 out]
                }
              }
              n238 = call "fgv_error_rc.vi"("cmd"=init-r-w."read") -> ("Error 2"=w449:T16)  [unwired: 10 in]
              n239 = Bundle By Name(cluster=w449, "제어단 특성변화"=w441) -> (w448:T16)
              n240 = call "fgv_error_rc.vi"("cmd"=init-r-w."write", "Error"=w448) -> ()  [unwired: 9 in, 1 out]
            }
            frame #1 {
              n241 = Unbundle By Name(w465) -> ("입력전류 RMS"=w462:dbl)
              n242 = Less Or Equal?(x=w462, y=w470) -> (x <= y?=w461:bool)
              n243 = Not A Number/Path/Refnum?(number/path/refnum=w462) -> (NaN/Path/Refnum?=w464:bool)
              n244 = Select(t=TRUE, s=w464, f=w461) -> (s? t:f=w460:bool)
              n245 = case shown="True" w460 {
                tunnel: w462 -> [_ w471]
                frame False {
                }
                frame True {
                  n246 = Number To Fractional String(number=w471) -> (F-format string=w472:string)  [unwired: 3 in]
                  n247 = call "fgv_status-display.vi"("Mode"=system-status."Update", "detail"=w472, "title"="Input RMS") -> ()  [unwired: 8 in, 1 out]
                }
              }
              n248 = case shown="True" w460 {
                tunnel: w470 -> [_ w475]
                frame False {
                }
                frame True {
                  n249 = Number To Fractional String(number=w475) -> (F-format string=w476:string)  [unwired: 3 in]
                  n250 = call "sub_log_basic.vi"("desc"=w476, "Title"="### DL950 input open") -> ()  [unwired: 9 in, 1 out]
                }
              }
              n251 = call "fgv_error_rc.vi"("cmd"=init-r-w."read") -> ("Error 2"=w468:T16)  [unwired: 10 in]
              n252 = Bundle By Name(cluster=w468, "제어단 단선"=w460) -> (w469:T16)
              n253 = call "fgv_error_rc.vi"("cmd"=init-r-w."write", "Error"=w469) -> ()  [unwired: 9 in, 1 out]
            }
            frame #2 {
              n254 = Unbundle By Name(w483) -> ("출력전류 RMS"=w480:dbl)
              n255 = In Range and Coerce(upper limit=w485, x=w480, lower limit=w484) -> (In Range?=w490:bool)  [unwired: 1 out]
              n256 = Not(x=w490) -> (.not. x?=w479:bool)
              n257 = Not A Number/Path/Refnum?(number/path/refnum=w480) -> (NaN/Path/Refnum?=w482:bool)
              n258 = Select(t=TRUE, s=w482, f=w479) -> (s? t:f=w478:bool)
              n259 = case shown="True" w478 {
                tunnel: w480 -> [_ w491]
                frame False {
                }
                frame True {
                  n260 = Number To Fractional String(number=w491) -> (F-format string=w492:string)  [unwired: 3 in]
                  n261 = call "fgv_status-display.vi"("Mode"=system-status."Update", "detail"=w492, "title"="Output RMS") -> ()  [unwired: 8 in, 1 out]
                }
              }
              n262 = case shown="True" w478 {
                tunnel: w480 -> [_ w495]
                frame False {
                }
                frame True {
                  n263 = Number To Fractional String(number=w495) -> (F-format string=w496:string)  [unwired: 3 in]
                  n264 = call "sub_log_basic.vi"("desc"=w496, "Title"="### DL950 output curr spec out ") -> ()  [unwired: 9 in, 1 out]
                }
              }
              n265 = call "fgv_error_rc.vi"("cmd"=init-r-w."read") -> ("Error 2"=w489:T16)  [unwired: 10 in]
              n266 = Bundle By Name(cluster=w489, "출력단 특성변화"=w478) -> (w488:T16)
              n267 = call "fgv_error_rc.vi"("cmd"=init-r-w."write", "Error"=w488) -> ()  [unwired: 9 in, 1 out]
            }
            frame #3 {
              n268 = Unbundle By Name(w503) -> ("출력전류 RMS"=w500:dbl)
              n269 = Less Or Equal?(x=w500, y=w504) -> (x <= y?=w499:bool)
              n270 = Not A Number/Path/Refnum?(number/path/refnum=w500) -> (NaN/Path/Refnum?=w502:bool)
              n271 = Select(t=TRUE, s=w502, f=w499) -> (s? t:f=w498:bool)
              n272 = case shown="True" w498 {
                tunnel: w500 -> [_ w509]
                frame False {
                }
                frame True {
                  n273 = Number To Fractional String(number=w509) -> (F-format string=w510:string)  [unwired: 3 in]
                  n274 = call "fgv_status-display.vi"("Mode"=system-status."Update", "detail"=w510, "title"="Output RMS") -> ()  [unwired: 8 in, 1 out]
                }
              }
              n275 = case shown="True" w498 {
                tunnel: w504 -> [_ w513]
                frame False {
                }
                frame True {
                  n276 = Number To Fractional String(number=w513) -> (F-format string=w514:string)  [unwired: 3 in]
                  n277 = call "sub_log_basic.vi"("desc"=w514, "Title"="### DL950 output open") -> ()  [unwired: 9 in, 1 out]
                }
              }
              n278 = call "fgv_error_rc.vi"("cmd"=init-r-w."read") -> ("Error 2"=w507:T16)  [unwired: 10 in]
              n279 = Bundle By Name(cluster=w507, "출력단 단선"=w498) -> (w508:T16)
              n280 = call "fgv_error_rc.vi"("cmd"=init-r-w."write", "Error"=w508) -> ()  [unwired: 9 in, 1 out]
            }
            frame #4 {
              n281 = Unbundle By Name(w522) -> ("온도"=w519:dbl)
              n282 = Not A Number/Path/Refnum?(number/path/refnum=w519) -> (NaN/Path/Refnum?=w521:bool)
              n283 = Less Or Equal?(x=w519, y=w523) -> (x <= y?=w518:bool)
              n284 = Not(x=w518) -> (.not. x?=w517:bool)
              n285 = Select(t=TRUE, s=w521, f=w517) -> (s? t:f=w516:bool)
              n286 = case shown="True" w516 {
                tunnel: w523 -> [_ w532]
                frame False {
                }
                frame True {
                  n287 = Number To Fractional String(number=w532) -> (F-format string=w533:string)  [unwired: 3 in]
                  n288 = call "sub_log_basic.vi"("desc"=w533, "Title"="### DL950 output open") -> ()  [unwired: 9 in, 1 out]
                }
              }
              n289 = case shown="True" w516 {
                tunnel: w519 -> [_ w528]
                frame False {
                }
                frame True {
                  n290 = Number To Fractional String(number=w528) -> (F-format string=w529:string)  [unwired: 3 in]
                  n291 = call "fgv_status-display.vi"("Mode"=system-status."Update", "detail"=w529, "title"="Temp") -> ()  [unwired: 8 in, 1 out]
                }
              }
              n292 = call "fgv_error_rc.vi"("cmd"=init-r-w."read") -> ("Error 2"=w526:T16)  [unwired: 10 in]
              n293 = Bundle By Name(cluster=w526, "온도"=w516) -> (w527:T16)
              n294 = call "fgv_error_rc.vi"("cmd"=init-r-w."write", "Error"=w527) -> ()  [unwired: 9 in, 1 out]
            }
            frame #5 {
              n295 = Unbundle By Name(w567) -> ("전압 63%[mS] Max"=w549:dbl, "전압 63%[mS] Min"=w548:dbl, "전압 98%[mS] Max"=w547:dbl, "전압 98%[mS] Min"=w546:dbl, "전류 37%[mS] Max"=w545:dbl, "전류 37%[mS] Min"=w544:dbl, "출력전류 Irms[mA] Max"=w543:dbl, "출력전류 Irms[mA] Min"=w542:dbl, "접촉저항[mOhm] Max"=w541:dbl, "접촉저항[mOhm] Min"=w540:dbl)
              n296 = Unbundle By Name(w568) -> ("입력카운트"=w550:dbl, "Rising Time 63%"=w565:dbl, "Rising Time 98%"=w564:dbl, "Failing Time 37%"=w563:dbl, "출력전류 RMS"=w562:dbl, "접촉저항"=w561:dbl, "방전전압"=w537:dbl)  [unwired: 1 out]
              n297 = Number To Decimal String(number=w551) -> (decimal integer string=w553:string)  [unwired: 1 in]
              n298 = call "fgv_rc-config.vi"("cmd"=rw."read") -> ("Testconfig out"=w538:T17)  [unwired: 9 in, 1 out]
              n299 = Unbundle By Name(w538) -> ("방전 기준[V]"=w536:dbl)
              n300 = call "sub_log_basic.vi"("desc"=w553, "Title"="input count") -> ()  [unwired: 9 in, 1 out]
              n301 = Build Array(w550, w565, w564, w563, w562, w561) -> (w560:dbl[])
              n302 = Less Or Equal?(x=w537, y=w536) -> (x <= y?=w535:bool)
              n303 = In Range and Coerce(upper limit=w549, x=w565, lower limit=w548) -> (In Range?=w559:bool)  [unwired: 1 out]
              n304 = In Range and Coerce(upper limit=w547, x=w564, lower limit=w546) -> (In Range?=w558:bool)  [unwired: 1 out]
              n305 = In Range and Coerce(upper limit=w545, x=w563, lower limit=w544) -> (In Range?=w557:bool)  [unwired: 1 out]
              n306 = In Range and Coerce(upper limit=w543, x=w562, lower limit=w542) -> (In Range?=w556:bool)  [unwired: 1 out]
              n307 = In Range and Coerce(upper limit=w541, x=w561, lower limit=w540) -> (In Range?=w555:bool)  [unwired: 1 out]
              n308 = Compound Arithmetic op=AND(w559, w558, w557, w556, w555, w535) -> (w554:bool)
              n309 = Build Array(w554, w559, w558, w557, w556, w555, w535) -> (w566:bool[])
              n310 = for {
                tunnel: w566 -> [w572] mode=indexing
                tunnel: w560 -> [w571] mode=indexing
                i -> [w570]
                n311 = Not(x=w572) -> (.not. x?=w569:bool)
                n312 = case shown="True" w569 {
                  tunnel: w571 -> [_ w577]
                  tunnel: w570 -> [_ w574]
                  frame False {
                  }
                  frame True {
                    n313 = Number To Fractional String(number=w577) -> (F-format string=w576:string)  [unwired: 3 in]
                    n314 = Index Array(array=string[] ["----------", "Rising Time 63%", "Rising Time 98%", "Failing Time 37%", "Output RMS", "Rcont"], index=w574) -> (element=w573:string)
                    n315 = call "fgv_status-display.vi"("Mode"=system-status."Update", "detail"=w576, "title"=w573) -> ()  [unwired: 8 in, 1 out]
                  }
                }
              }
            }
            frame #6 {
              # "디스플레이"
              n316 = Unbundle By Name(w594) -> ("입력카운트"=w588:dbl)
              n317 = Cluster To Array(cluster=w594) -> (array=w613:dbl[])
              n318 = To Long Integer(number=w585) -> (32bit integer=w583:i32)
              n319 = To Double Precision Float(number=w615) -> (double precision float=w612:dbl)
              n320 = Split 1D Array(array=w613, index=2) -> (second subarray=w611:dbl[])  [unwired: 1 out]
              n321 = Increment(x=w612) -> ()  [unwired: 1 out]
              n322 = call "fgv_error_rc.vi"("cmd"=init-r-w."read") -> ("Error 2"=w624:T16)  [unwired: 10 in]
              n323 = Unbundle By Name(w624) -> ("제어단 단선"=w623:bool, "제어단 단락"=w622:bool, "제어단 특성변화"=w621:bool, "출력단 단선"=w620:bool, "출력단 단락"=w619:bool, "출력단 특성변화"=w618:bool, "온도"=w617:bool)
              n324 = And Array Elements(Boolean array=w593) -> (logical AND=w592:bool)
              n325 = Select(t=w588, s=w592, f=0.0) -> (s? t:f=w587:dbl)
              n326 = Build Array(w588, w587) -> (w586:dbl[])
              n327 = Build Array(w623, w622, w621, w620, w619, w618, w617) -> (w610:bool[])
              n328 = call "count_run 1.vi"("cmd"=cmd_count."count", "CH"=w583, "Array_Count"=w586) -> ("Array_data"=w584:dbl[][])  [unwired: 7 in, 1 out]
              n329 = Not(x=w610) -> (.not. x?=w627:bool[])
              n330 = Index Array(array=w584, index (row)=w583) -> (element=w582:dbl[])  [unwired: 1 in]
              n331 = Index Array(array=w582) -> (element #1=w581:dbl, element #2=w580:dbl)  [unwired: 2 in]
              n332 = Build Array (concatenate)(w593, w627) -> (w596:bool[])
              n333 = Build Array (concatenate)(w581, w580, w611) -> (w579:dbl[])
              n334 = for {
                tunnel: w596 -> [w662] mode=indexing
                tunnel: [w659] -> w609 mode=indexing
                n335 = Select(t="OK", s=w662, f="NG") -> (s? t:f=w659:string)
              }
              n336 = Split 1D Array(array=w579, index=14) -> (first subarray=w625:dbl[])  [unwired: 1 out]
              n337 = And Array Elements(Boolean array=w596) -> (logical AND=w597:bool)
              n338 = for {
                tunnel: w625 -> [w633] mode=indexing
                tunnel: [w632] -> w600 mode=indexing
                tunnel: i16[] [0, 0, 0, 1, 1, 1, 1, 1, 1, 3, 1, 1, 1, 1] -> [w631] mode=indexing
                n339 = Number To Fractional String(number=w633, precision (6)=w631) -> (F-format string=w632:string)  [unwired: 2 in]
              }
              n340 = case shown="False" w597 {
                tunnel: w597 -> [w649 _]
                tunnel: w596 -> [w648 _]
                frame False {
                  n341 = call "sub_shutdown.vi"("type"=shutdown-type."all") -> ()  [unwired: 10 in, 1 out]
                  n342 = for {
                    tunnel: w649 -> [w654]
                    tunnel: string[] ["제어단 단선", "제어단 단락", "제어단특성변화", "출력단 단선", "출력단 단락", "출력단 특성변화", "온도"] -> [w653]
                    tunnel: w648 -> [_] mode=indexing
                    i -> [w652]
                    n343 = case shown="True" w654 {
                      tunnel: w653 -> [_ w657]
                      tunnel: w652 -> [_ w656]
                      frame False {
                      }
                      frame True {
                        n344 = Index Array(array=w657, index=w656) -> (element=w655:string)
                        n345 = call "sub_log_basic.vi"("desc"=w655, "Title"="Shutdown ") -> ()  [unwired: 9 in, 1 out]
                      }
                    }
                  }
                }
                frame True {
                }
              }
              n346 = Build Array (concatenate)(w600, w609) -> (w598:string[])
              n347 = call "fgv_error_rc.vi"("cmd"=init-r-w."read") -> ("Error 2"=w607:T16)  [unwired: 10 in]
              n348 = Unbundle By Name(w607) -> ("제어단 단락"=w604:bool, "출력단 단락"=w603:bool)
              n349 = Array Size(array=w598) -> (size(s)=w605:i32)
              n350 = Initialize Array("-", w605) -> (w601:string[])
              n351 = Or(x=w604, y=w603) -> (x .or. y?=w602:bool)
              n352 = Select(t=w601, s=w602, f=w598) -> (s? t:f=w599:string[])
              n353 = case shown="True" w602 {
                tunnel: [w634 w645] -> w595
                tunnel: w599 -> [w634 w647]
                tunnel: w604 -> [_ w643]
                tunnel: w603 -> [_ w635]
                frame False {
                }
                frame True {
                  n354 = Select(t="NG", s=w643, f="OK") -> (s? t:f=w640:string)
                  n355 = Replace Array Subset(array=w647, new element=w640, index=20) -> (w646:string[])
                  n356 = Select(t="NG", s=w635, f="OK") -> (s? t:f=w636:string)
                  n357 = Replace Array Subset(array=w646, new element=w636, index=23) -> (w645:string[])
                }
              }
              n358 = call "TableCnt.vi"("cnt"=cmd_tablecnt."Write", "appended array"=w595) -> ()  [unwired: 8 in, 2 out]
              n359 = disable-structure shown="Disabled" {
                disable-tunnel: w595 -> [w629 _]
                frame Disabled {
                  n360 = call "fgv_ngok_global.vi"("cmd"=rw."write", "results"=w629) -> ()  [unwired: 9 in, 1 out]
                }
                frame Enabled {
                }
              }
            }
            frame #7 {
            }
          }
        }
        frame "B2" {
          n361 = call "fgv_judgement.vi"("cmd"=rw."read") -> ("Test Judgement 2"=w666:T20)  [unwired: 9 in, 1 out]
          n362 = call "fgv_measure_reg.vi"("cmd"=rw."read") -> ("measure_reg 2"=w663:T21)  [unwired: 10 in]
          n363 = stacked-sequence {
            seq-local: [_ _ _ _ _ w786 _ _] -> [_ _ _ _ _ _ w840 _]
            tunnel: w675 -> [w688 _ _ _ _ _ _ _]
            tunnel: w674 -> [w687 _ _ _ _ _ _ _]
            tunnel: w673 -> [_ w706 _ _ _ _ _ _]
            tunnel: w672 -> [_ _ w721 _ _ _ _ _]
            tunnel: w671 -> [_ _ w720 _ _ _ _ _]
            tunnel: w670 -> [_ _ _ w740 _ _ _ _]
            tunnel: w669 -> [_ _ _ _ w759 _ _ _]
            tunnel: w668 -> [_ _ _ _ _ w795 _ _]
            tunnel: w666 -> [_ _ _ _ _ w794 _ _]
            tunnel: w665 -> [_ _ _ _ _ _ w800 w872]
            tunnel: w663 -> [w681 w701 w719 w739 w758 w793 w836 _]
            frame #0 {
              n364 = Unbundle By Name(w681) -> ("입력전류 RMS"=w678:dbl)
              n365 = In Range and Coerce(upper limit=w688, x=w678, lower limit=w687) -> (In Range?=w686:bool)  [unwired: 1 out]
              n366 = Not(x=w686) -> (.not. x?=w677:bool)
              n367 = Not A Number/Path/Refnum?(number/path/refnum=w678) -> (NaN/Path/Refnum?=w680:bool)
              n368 = Select(t=TRUE, s=w680, f=w677) -> (s? t:f=w676:bool)
              n369 = case shown="True" w676 {
                tunnel: w678 -> [_ w693]
                frame False {
                }
                frame True {
                  n370 = Number To Fractional String(number=w693) -> (F-format string=w694:string)  [unwired: 3 in]
                  n371 = call "sub_log_basic.vi"("desc"=w694, "Title"="### DL950 input curr spec out ") -> ()  [unwired: 9 in, 1 out]
                }
              }
              n372 = case shown="True" w676 {
                tunnel: w678 -> [_ w689]
                frame False {
                }
                frame True {
                  n373 = Number To Fractional String(number=w689) -> (F-format string=w690:string)  [unwired: 3 in]
                  n374 = call "fgv_status-display.vi"("Mode"=system-status."Update", "detail"=w690, "title"="Input RMS") -> ()  [unwired: 8 in, 1 out]
                }
              }
              n375 = call "fgv_error_rc.vi"("cmd"=init-r-w."read") -> ("Error 2"=w685:T16)  [unwired: 10 in]
              n376 = Bundle By Name(cluster=w685, "제어단 특성변화"=w676) -> (w684:T16)
              n377 = call "fgv_error_rc.vi"("cmd"=init-r-w."write", "Error"=w684) -> ()  [unwired: 9 in, 1 out]
            }
            frame #1 {
              n378 = Unbundle By Name(w701) -> ("입력전류 RMS"=w698:dbl)
              n379 = Less Or Equal?(x=w698, y=w706) -> (x <= y?=w697:bool)
              n380 = Not A Number/Path/Refnum?(number/path/refnum=w698) -> (NaN/Path/Refnum?=w700:bool)
              n381 = Select(t=TRUE, s=w700, f=w697) -> (s? t:f=w696:bool)
              n382 = call "fgv_error_rc.vi"("cmd"=init-r-w."read") -> ("Error 2"=w704:T16)  [unwired: 10 in]
              n383 = Bundle By Name(cluster=w704, "제어단 단선"=w696) -> (w705:T16)
              n384 = case shown="True" w696 {
                tunnel: w706 -> [_ w711]
                frame False {
                }
                frame True {
                  n385 = Number To Fractional String(number=w711) -> (F-format string=w712:string)  [unwired: 3 in]
                  n386 = call "sub_log_basic.vi"("desc"=w712, "Title"="### DL950 input open") -> ()  [unwired: 9 in, 1 out]
                }
              }
              n387 = case shown="True" w696 {
                tunnel: w698 -> [_ w707]
                frame False {
                }
                frame True {
                  n388 = Number To Fractional String(number=w707) -> (F-format string=w708:string)  [unwired: 3 in]
                  n389 = call "fgv_status-display.vi"("Mode"=system-status."Update", "detail"=w708, "title"="Input RMS") -> ()  [unwired: 8 in, 1 out]
                }
              }
              n390 = call "fgv_error_rc.vi"("cmd"=init-r-w."write", "Error"=w705) -> ()  [unwired: 9 in, 1 out]
            }
            frame #2 {
              n391 = Unbundle By Name(w719) -> ("출력전류 RMS"=w716:dbl)
              n392 = In Range and Coerce(upper limit=w721, x=w716, lower limit=w720) -> (In Range?=w726:bool)  [unwired: 1 out]
              n393 = Not(x=w726) -> (.not. x?=w715:bool)
              n394 = Not A Number/Path/Refnum?(number/path/refnum=w716) -> (NaN/Path/Refnum?=w718:bool)
              n395 = Select(t=TRUE, s=w718, f=w715) -> (s? t:f=w714:bool)
              n396 = case shown="True" w714 {
                tunnel: w716 -> [_ w731]
                frame False {
                }
                frame True {
                  n397 = Number To Fractional String(number=w731) -> (F-format string=w732:string)  [unwired: 3 in]
                  n398 = call "sub_log_basic.vi"("desc"=w732, "Title"="### DL950 output curr spec out ") -> ()  [unwired: 9 in, 1 out]
                }
              }
              n399 = case shown="True" w714 {
                tunnel: w716 -> [_ w727]
                frame False {
                }
                frame True {
                  n400 = Number To Fractional String(number=w727) -> (F-format string=w728:string)  [unwired: 3 in]
                  n401 = call "fgv_status-display.vi"("Mode"=system-status."Update", "detail"=w728, "title"="Output RMS") -> ()  [unwired: 8 in, 1 out]
                }
              }
              n402 = call "fgv_error_rc.vi"("cmd"=init-r-w."read") -> ("Error 2"=w725:T16)  [unwired: 10 in]
              n403 = Bundle By Name(cluster=w725, "출력단 특성변화"=w714) -> (w724:T16)
              n404 = call "fgv_error_rc.vi"("cmd"=init-r-w."write", "Error"=w724) -> ()  [unwired: 9 in, 1 out]
            }
            frame #3 {
              n405 = Unbundle By Name(w739) -> ("출력전류 RMS"=w735:dbl)
              n406 = Less Or Equal?(x=w735, y=w740) -> (x <= y?=w736:bool)
              n407 = Not A Number/Path/Refnum?(number/path/refnum=w735) -> (NaN/Path/Refnum?=w738:bool)
              n408 = Select(t=TRUE, s=w738, f=w736) -> (s? t:f=w734:bool)
              n409 = case shown="True" w734 {
                tunnel: w740 -> [_ w749]
                frame False {
                }
                frame True {
                  n410 = Number To Fractional String(number=w749) -> (F-format string=w750:string)  [unwired: 3 in]
                  n411 = call "sub_log_basic.vi"("desc"=w750, "Title"="### DL950 output open") -> ()  [unwired: 9 in, 1 out]
                }
              }
              n412 = case shown="True" w734 {
                tunnel: w735 -> [_ w745]
                frame False {
                }
                frame True {
                  n413 = Number To Fractional String(number=w745) -> (F-format string=w746:string)  [unwired: 3 in]
                  n414 = call "fgv_status-display.vi"("Mode"=system-status."Update", "detail"=w746, "title"="Output RMS") -> ()  [unwired: 8 in, 1 out]
                }
              }
              n415 = call "fgv_error_rc.vi"("cmd"=init-r-w."read") -> ("Error 2"=w743:T16)  [unwired: 10 in]
              n416 = Bundle By Name(cluster=w743, "출력단 단선"=w734) -> (w744:T16)
              n417 = call "fgv_error_rc.vi"("cmd"=init-r-w."write", "Error"=w744) -> ()  [unwired: 9 in, 1 out]
            }
            frame #4 {
              n418 = Unbundle By Name(w758) -> ("온도"=w755:dbl)
              n419 = Less Or Equal?(x=w755, y=w759) -> (x <= y?=w754:bool)
              n420 = Not(x=w754) -> (.not. x?=w753:bool)
              n421 = Not A Number/Path/Refnum?(number/path/refnum=w755) -> (NaN/Path/Refnum?=w757:bool)
              n422 = Select(t=TRUE, s=w757, f=w753) -> (s? t:f=w752:bool)
              n423 = case shown="True" w752 {
                tunnel: w759 -> [_ w768]
                frame False {
                }
                frame True {
                  n424 = Number To Fractional String(number=w768) -> (F-format string=w769:string)  [unwired: 3 in]
                  n425 = call "sub_log_basic.vi"("desc"=w769, "Title"="### DL950 output open") -> ()  [unwired: 9 in, 1 out]
                }
              }
              n426 = case shown="True" w752 {
                tunnel: w755 -> [_ w764]
                frame False {
                }
                frame True {
                  n427 = Number To Fractional String(number=w764) -> (F-format string=w765:string)  [unwired: 3 in]
                  n428 = call "fgv_status-display.vi"("Mode"=system-status."Update", "detail"=w765, "title"="온도") -> ()  [unwired: 8 in, 1 out]
                }
              }
              n429 = call "fgv_error_rc.vi"("cmd"=init-r-w."read") -> ("Error 2"=w762:T16)  [unwired: 10 in]
              n430 = Bundle By Name(cluster=w762, "온도"=w752) -> (w763:T16)
              n431 = call "fgv_error_rc.vi"("cmd"=init-r-w."write", "Error"=w763) -> ()  [unwired: 9 in, 1 out]
            }
            frame #5 {
              n432 = Unbundle By Name(w794) -> ("출력전류 Irms[mA] Max"=w772:dbl, "출력전류 Irms[mA] Min"=w771:dbl)
              n433 = Unbundle By Name(w793) -> ("입력카운트"=w782:dbl, "출력카운트"=w778:dbl, "출력전류 RMS"=w775:dbl)
              n434 = To Double Precision Float(number=w795) -> ()  [unwired: 1 out]
              n435 = Equal?(x=w782, y=w778) -> (x = y?=w792:bool)
              n436 = In Range and Coerce(upper limit=w772, x=w775, lower limit=w771) -> (In Range?=w791:bool)  [unwired: 1 out]
              n437 = Build Array(w792, w791) -> (w786:bool[])
              n438 = Number To Fractional String(number=w775) -> (F-format string=w774:string)  [unwired: 3 in]
              n439 = call "sub_log_basic.vi"("desc"=w774, "Title"="출력전류") -> ("error out"=w773:errorcluster)  [unwired: 9 in]
              n440 = Number To Decimal String(number=w782) -> (decimal integer string=w781:string)  [unwired: 1 in]
              n441 = call "sub_log_basic.vi"("error in"=w773, "desc"=w781, "Title"="입력 카운트") -> ("error out"=w777:errorcluster)  [unwired: 8 in]
              n442 = Number To Decimal String(number=w778) -> (decimal integer string=w780:string)  [unwired: 1 in]
              n443 = call "sub_log_basic.vi"("error in"=w777, "desc"=w780, "Title"="출력 카운트") -> ()  [unwired: 8 in, 1 out]
              n444 = Not(x=w786) -> (.not. x?=w784:bool[])
              n445 = Array To Cluster(array=w784) -> (cluster=w785:cluster{"[0]":bool, "[1]":bool})
              n446 = call "fgv_curr-test-info.vi"("cmd"=rw."read") -> ("현재테스트 정보 2"=w788:T4)  [unwired: 10 in]
              n447 = Bundle By Name(cluster=w788, "NG"=w785) -> (w787:T4)
              n448 = call "fgv_curr-test-info.vi"("cmd"=rw."write", "현재테스트 정보"=w787) -> ()  [unwired: 9 in, 1 out]
            }
            frame #6 {
              # "디스플레이"
              n449 = Cluster To Array(cluster=w836) -> (array=w801:dbl[])
              n450 = To Long Integer(number=w800) -> (32bit integer=w799:i32)
              n451 = Index Array(array=w801) -> (element #1=w808:dbl, element #2=w807:dbl)  [unwired: 2 in]
              n452 = Build Array(w808, w807) -> (w811:dbl[])
              n453 = call "fgv_error_rc.vi"("cmd"=init-r-w."read") -> ("Error 2"=w827:T16)  [unwired: 10 in]
              n454 = call "count_run 1.vi"("cmd"=cmd_count."count", "CH"=w799, "Array_Count"=w811) -> ("Array_data"=w810:dbl[][])  [unwired: 7 in, 1 out]
              n455 = Unbundle By Name(w827) -> ("제어단 단선"=w835:bool, "제어단 단락"=w834:bool, "제어단 특성변화"=w833:bool, "출력단 단선"=w832:bool, "출력단 단락"=w831:bool, "출력단 특성변화"=w830:bool, "온도"=w829:bool)
              n456 = Index Array(array=w810, index (row)=w799) -> (element=w809:dbl[])  [unwired: 1 in]
              n457 = Index Array(array=w809) -> (element #1=w805:dbl, element #2=w802:dbl)  [unwired: 2 in]
              n458 = Replace Array Subset(array=w801, new element=w805, index=0) -> (w803:dbl[])
              n459 = Build Array(w835, w834, w833, w832, w831, w830, w829) -> (w825:bool[])
              n460 = Not(x=w840) -> (.not. x?=w826:bool[])
              n461 = Replace Array Subset(array=w803, new element=w802, index=1) -> (w797:dbl[])
              n462 = Build Array (concatenate)(w826, w825) -> (w813:bool[])
              n463 = Or Array Elements(Boolean array=w813) -> (logical OR=w837:bool)
              n464 = for {
                tunnel: [w843] -> w796 mode=indexing
                tunnel: w797 -> [w842] mode=indexing
                tunnel: i16[] [0, 0, 1, 1, 1, 1, 1] -> [w841] mode=indexing
                n465 = Number To Fractional String(number=w842, precision (6)=w841) -> (F-format string=w843:string)  [unwired: 2 in]
              }
              n466 = case shown="True" w837 {
                tunnel: w813 -> [_ w859]
                frame False {
                }
                frame True {
                  n467 = call "sub_shutdown.vi"("type"=shutdown-type."all") -> ()  [unwired: 10 in, 1 out]
                  n468 = for {
                    tunnel: w859 -> [w863] mode=indexing
                    tunnel: string[] ["제어단 단선", "제어단 단락", "제어단특성변화", "출력단 단선", "출력단 단락", "출력단 특성변화", "온도"] -> [w862]
                    i -> [w861]
                    n469 = case shown="True" w863 {
                      tunnel: w862 -> [_ w866]
                      tunnel: w861 -> [_ w865]
                      frame False {
                      }
                      frame True {
                        n470 = Index Array(array=w866, index=w865) -> (element=w864:string)
                        n471 = call "sub_log_basic.vi"("desc"=w864, "Title"="Shutdown ") -> ()  [unwired: 9 in, 1 out]
                      }
                    }
                  }
                }
              }
              n472 = for {
                tunnel: w813 -> [w871] mode=indexing
                tunnel: [w868] -> w839 mode=indexing
                n473 = Select(t="NG", s=w871, f="OK") -> (s? t:f=w868:string)
              }
              n474 = Build Array (concatenate)(w796, w839) -> (w815:string[])
              n475 = call "fgv_error_rc.vi"("cmd"=init-r-w."read") -> ("Error 2"=w823:T16)  [unwired: 10 in]
              n476 = Unbundle By Name(w823) -> ("제어단 단락"=w820:bool, "출력단 단락"=w819:bool)
              n477 = Array Size(array=w815) -> (size(s)=w821:i32)
              n478 = Initialize Array("-", w821) -> (w817:string[])
              n479 = Or(x=w820, y=w819) -> (x .or. y?=w818:bool)
              n480 = Select(t=w817, s=w818, f=w815) -> (s? t:f=w816:string[])
              n481 = case shown="True" w818 {
                tunnel: [w844 w855] -> w814
                tunnel: w816 -> [w844 w857]
                tunnel: w820 -> [_ w853]
                tunnel: w819 -> [_ w845]
                frame False {
                }
                frame True {
                  n482 = Select(t="NG", s=w853, f="OK") -> (s? t:f=w850:string)
                  n483 = Replace Array Subset(array=w857, new element=w850, index=9) -> (w856:string[])
                  n484 = Select(t="NG", s=w845, f="OK") -> (s? t:f=w846:string)
                  n485 = Replace Array Subset(array=w856, new element=w846, index=12) -> (w855:string[])
                }
              }
              n486 = call "TableCnt.vi"("cnt"=cmd_tablecnt."Write", "appended array"=w814) -> ()  [unwired: 8 in, 2 out]
            }
            frame #7 {
              # "저장"
              n487 = call "TableCnt.vi"("cnt"=cmd_tablecnt."Default") -> ("Item Names"=w873:string[][])  [unwired: 9 in, 1 out]
              n488 = Index Array(array=w873, index (col)=w872) -> ()  [unwired: 1 in, 1 out]
            }
          }
        }
        frame "B3" {
          n489 = call "fgv_judgement.vi"("cmd"=rw."read") -> ("Test Judgement 2"=w878:T20)  [unwired: 9 in, 1 out]
          n490 = call "fgv_measure_reg.vi"("cmd"=rw."read") -> ("measure_reg 2"=w875:T21)  [unwired: 10 in]
          n491 = stacked-sequence {
            seq-local: [_ _ _ _ _ w998 _ _] -> [_ _ _ _ _ _ w1052 _]
            tunnel: w887 -> [w900 _ _ _ _ _ _ _]
            tunnel: w886 -> [w899 _ _ _ _ _ _ _]
            tunnel: w885 -> [_ w918 _ _ _ _ _ _]
            tunnel: w884 -> [_ _ w933 _ _ _ _ _]
            tunnel: w883 -> [_ _ w932 _ _ _ _ _]
            tunnel: w882 -> [_ _ _ w952 _ _ _ _]
            tunnel: w881 -> [_ _ _ _ w971 _ _ _]
            tunnel: w880 -> [_ _ _ _ _ w1007 _ _]
            tunnel: w878 -> [_ _ _ _ _ w1006 _ _]
            tunnel: w877 -> [_ _ _ _ _ _ w1017 w1084]
            tunnel: w875 -> [w893 w913 w931 w951 w970 w1005 w1047 _]
            frame #0 {
              n492 = Unbundle By Name(w893) -> ("입력전류 RMS"=w890:dbl)
              n493 = In Range and Coerce(upper limit=w900, x=w890, lower limit=w899) -> (In Range?=w898:bool)  [unwired: 1 out]
              n494 = Not(x=w898) -> (.not. x?=w889:bool)
              n495 = Not A Number/Path/Refnum?(number/path/refnum=w890) -> (NaN/Path/Refnum?=w892:bool)
              n496 = Select(t=TRUE, s=w892, f=w889) -> (s? t:f=w888:bool)
              n497 = case shown="True" w888 {
                tunnel: w890 -> [_ w905]
                frame False {
                }
                frame True {
                  n498 = Number To Fractional String(number=w905) -> (F-format string=w906:string)  [unwired: 3 in]
                  n499 = call "sub_log_basic.vi"("desc"=w906, "Title"="### DL950 input curr spec out ") -> ()  [unwired: 9 in, 1 out]
                }
              }
              n500 = case shown="True" w888 {
                tunnel: w890 -> [_ w901]
                frame False {
                }
                frame True {
                  n501 = Number To Fractional String(number=w901) -> (F-format string=w902:string)  [unwired: 3 in]
                  n502 = call "fgv_status-display.vi"("Mode"=system-status."Update", "detail"=w902, "title"="Input RMS") -> ()  [unwired: 8 in, 1 out]
                }
              }
              n503 = call "fgv_error_rc.vi"("cmd"=init-r-w."read") -> ("Error 2"=w897:T16)  [unwired: 10 in]
              n504 = Bundle By Name(cluster=w897, "제어단 특성변화"=w888) -> (w896:T16)
              n505 = call "fgv_error_rc.vi"("cmd"=init-r-w."write", "Error"=w896) -> ()  [unwired: 9 in, 1 out]
            }
            frame #1 {
              n506 = Unbundle By Name(w913) -> ("입력전류 RMS"=w910:dbl)
              n507 = Less Or Equal?(x=w910, y=w918) -> (x <= y?=w909:bool)
              n508 = Not A Number/Path/Refnum?(number/path/refnum=w910) -> (NaN/Path/Refnum?=w912:bool)
              n509 = Select(t=TRUE, s=w912, f=w909) -> (s? t:f=w908:bool)
              n510 = call "fgv_error_rc.vi"("cmd"=init-r-w."read") -> ("Error 2"=w916:T16)  [unwired: 10 in]
              n511 = Bundle By Name(cluster=w916, "제어단 단선"=w908) -> (w917:T16)
              n512 = case shown="True" w908 {
                tunnel: w918 -> [_ w923]
                frame False {
                }
                frame True {
                  n513 = Number To Fractional String(number=w923) -> (F-format string=w924:string)  [unwired: 3 in]
                  n514 = call "sub_log_basic.vi"("desc"=w924, "Title"="### DL950 input open") -> ()  [unwired: 9 in, 1 out]
                }
              }
              n515 = case shown="True" w908 {
                tunnel: w910 -> [_ w919]
                frame False {
                }
                frame True {
                  n516 = Number To Fractional String(number=w919) -> (F-format string=w920:string)  [unwired: 3 in]
                  n517 = call "fgv_status-display.vi"("Mode"=system-status."Update", "detail"=w920, "title"="Input RMS") -> ()  [unwired: 8 in, 1 out]
                }
              }
              n518 = call "fgv_error_rc.vi"("cmd"=init-r-w."write", "Error"=w917) -> ()  [unwired: 9 in, 1 out]
            }
            frame #2 {
              n519 = Unbundle By Name(w931) -> ("출력전류 RMS"=w928:dbl)
              n520 = In Range and Coerce(upper limit=w933, x=w928, lower limit=w932) -> (In Range?=w938:bool)  [unwired: 1 out]
              n521 = Not(x=w938) -> (.not. x?=w927:bool)
              n522 = Not A Number/Path/Refnum?(number/path/refnum=w928) -> (NaN/Path/Refnum?=w930:bool)
              n523 = Select(t=TRUE, s=w930, f=w927) -> (s? t:f=w926:bool)
              n524 = case shown="True" w926 {
                tunnel: w928 -> [_ w943]
                frame False {
                }
                frame True {
                  n525 = Number To Fractional String(number=w943) -> (F-format string=w944:string)  [unwired: 3 in]
                  n526 = call "sub_log_basic.vi"("desc"=w944, "Title"="### DL950 output curr spec out ") -> ()  [unwired: 9 in, 1 out]
                }
              }
              n527 = case shown="True" w926 {
                tunnel: w928 -> [_ w939]
                frame False {
                }
                frame True {
                  n528 = Number To Fractional String(number=w939) -> (F-format string=w940:string)  [unwired: 3 in]
                  n529 = call "fgv_status-display.vi"("Mode"=system-status."Update", "detail"=w940, "title"="Output RMS") -> ()  [unwired: 8 in, 1 out]
                }
              }
              n530 = call "fgv_error_rc.vi"("cmd"=init-r-w."read") -> ("Error 2"=w937:T16)  [unwired: 10 in]
              n531 = Bundle By Name(cluster=w937, "출력단 특성변화"=w926) -> (w936:T16)
              n532 = call "fgv_error_rc.vi"("cmd"=init-r-w."write", "Error"=w936) -> ()  [unwired: 9 in, 1 out]
            }
            frame #3 {
              n533 = Unbundle By Name(w951) -> ("출력전류 RMS"=w947:dbl)
              n534 = Less Or Equal?(x=w947, y=w952) -> (x <= y?=w948:bool)
              n535 = Not A Number/Path/Refnum?(number/path/refnum=w947) -> (NaN/Path/Refnum?=w950:bool)
              n536 = Select(t=TRUE, s=w950, f=w948) -> (s? t:f=w946:bool)
              n537 = case shown="True" w946 {
                tunnel: w952 -> [_ w961]
                frame False {
                }
                frame True {
                  n538 = Number To Fractional String(number=w961) -> (F-format string=w962:string)  [unwired: 3 in]
                  n539 = call "sub_log_basic.vi"("desc"=w962, "Title"="### DL950 output open") -> ()  [unwired: 9 in, 1 out]
                }
              }
              n540 = case shown="True" w946 {
                tunnel: w947 -> [_ w957]
                frame False {
                }
                frame True {
                  n541 = Number To Fractional String(number=w957) -> (F-format string=w958:string)  [unwired: 3 in]
                  n542 = call "fgv_status-display.vi"("Mode"=system-status."Update", "detail"=w958, "title"="Output RMS") -> ()  [unwired: 8 in, 1 out]
                }
              }
              n543 = call "fgv_error_rc.vi"("cmd"=init-r-w."read") -> ("Error 2"=w955:T16)  [unwired: 10 in]
              n544 = Bundle By Name(cluster=w955, "출력단 단선"=w946) -> (w956:T16)
              n545 = call "fgv_error_rc.vi"("cmd"=init-r-w."write", "Error"=w956) -> ()  [unwired: 9 in, 1 out]
            }
            frame #4 {
              n546 = Unbundle By Name(w970) -> ("온도"=w967:dbl)
              n547 = Less Or Equal?(x=w967, y=w971) -> (x <= y?=w966:bool)
              n548 = Not(x=w966) -> (.not. x?=w965:bool)
              n549 = Not A Number/Path/Refnum?(number/path/refnum=w967) -> (NaN/Path/Refnum?=w969:bool)
              n550 = Select(t=TRUE, s=w969, f=w965) -> (s? t:f=w964:bool)
              n551 = case shown="True" w964 {
                tunnel: w971 -> [_ w980]
                frame False {
                }
                frame True {
                  n552 = Number To Fractional String(number=w980) -> (F-format string=w981:string)  [unwired: 3 in]
                  n553 = call "sub_log_basic.vi"("desc"=w981, "Title"="### DL950 output open") -> ()  [unwired: 9 in, 1 out]
                }
              }
              n554 = case shown="True" w964 {
                tunnel: w967 -> [_ w976]
                frame False {
                }
                frame True {
                  n555 = Number To Fractional String(number=w976) -> (F-format string=w977:string)  [unwired: 3 in]
                  n556 = call "fgv_status-display.vi"("Mode"=system-status."Update", "detail"=w977, "title"="온도") -> ()  [unwired: 8 in, 1 out]
                }
              }
              n557 = call "fgv_error_rc.vi"("cmd"=init-r-w."read") -> ("Error 2"=w974:T16)  [unwired: 10 in]
              n558 = Bundle By Name(cluster=w974, "온도"=w964) -> (w975:T16)
              n559 = call "fgv_error_rc.vi"("cmd"=init-r-w."write", "Error"=w975) -> ()  [unwired: 9 in, 1 out]
            }
            frame #5 {
              n560 = Unbundle By Name(w1006) -> ("출력전류 Irms[mA] Max"=w984:dbl, "출력전류 Irms[mA] Min"=w983:dbl)
              n561 = Unbundle By Name(w1005) -> ("입력카운트"=w994:dbl, "출력카운트"=w990:dbl, "출력전류 RMS"=w987:dbl)
              n562 = To Double Precision Float(number=w1007) -> ()  [unwired: 1 out]
              n563 = Equal?(x=w994, y=w990) -> (x = y?=w1004:bool)
              n564 = In Range and Coerce(upper limit=w984, x=w987, lower limit=w983) -> (In Range?=w1003:bool)  [unwired: 1 out]
              n565 = Build Array(w1004, w1003) -> (w998:bool[])
              n566 = Number To Fractional String(number=w987) -> (F-format string=w986:string)  [unwired: 3 in]
              n567 = call "sub_log_basic.vi"("desc"=w986, "Title"="출력전류") -> ("error out"=w985:errorcluster)  [unwired: 9 in]
              n568 = Number To Decimal String(number=w994) -> (decimal integer string=w993:string)  [unwired: 1 in]
              n569 = call "sub_log_basic.vi"("error in"=w985, "desc"=w993, "Title"="입력 카운트") -> ("error out"=w989:errorcluster)  [unwired: 8 in]
              n570 = Number To Decimal String(number=w990) -> (decimal integer string=w992:string)  [unwired: 1 in]
              n571 = call "sub_log_basic.vi"("error in"=w989, "desc"=w992, "Title"="출력 카운트") -> ()  [unwired: 8 in, 1 out]
              n572 = Not(x=w998) -> (.not. x?=w996:bool[])
              n573 = Array To Cluster(array=w996) -> (cluster=w997:cluster{"[0]":bool, "[1]":bool})
              n574 = call "fgv_curr-test-info.vi"("cmd"=rw."read") -> ("현재테스트 정보 2"=w1000:T4)  [unwired: 10 in]
              n575 = Bundle By Name(cluster=w1000, "NG"=w997) -> (w999:T4)
              n576 = call "fgv_curr-test-info.vi"("cmd"=rw."write", "현재테스트 정보"=w999) -> ()  [unwired: 9 in, 1 out]
            }
            frame #6 {
              # "디스플레이"
              n577 = To Long Integer(number=w1017) -> (32bit integer=w1016:i32)
              n578 = Cluster To Array(cluster=w1047) -> (array=w1015:dbl[])
              n579 = Index Array(array=w1015) -> (element #1=w1019:dbl, element #2=w1018:dbl)  [unwired: 2 in]
              n580 = call "fgv_error_rc.vi"("cmd"=init-r-w."read") -> ("Error 2"=w1038:T16)  [unwired: 10 in]
              n581 = Build Array(w1019, w1018) -> (w1022:dbl[])
              n582 = Unbundle By Name(w1038) -> ("제어단 단선"=w1046:bool, "제어단 단락"=w1045:bool, "제어단 특성변화"=w1044:bool, "출력단 단선"=w1043:bool, "출력단 단락"=w1042:bool, "출력단 특성변화"=w1041:bool, "온도"=w1040:bool)
              n583 = call "count_run 1.vi"("cmd"=cmd_count."count", "CH"=w1016, "Array_Count"=w1022) -> ("Array_data"=w1021:dbl[][])  [unwired: 7 in, 1 out]
              n584 = Index Array(array=w1021, index (row)=w1016) -> (element=w1020:dbl[])  [unwired: 1 in]
              n585 = Index Array(array=w1020) -> (element #1=w1013:dbl, element #2=w1010:dbl)  [unwired: 2 in]
              n586 = Replace Array Subset(array=w1015, new element=w1013, index=0) -> (w1011:dbl[])
              n587 = Build Array(w1046, w1045, w1044, w1043, w1042, w1041, w1040) -> (w1036:bool[])
              n588 = Not(x=w1052) -> (.not. x?=w1037:bool[])
              n589 = Replace Array Subset(array=w1011, new element=w1010, index=1) -> (w1009:dbl[])
              n590 = Build Array (concatenate)(w1037, w1036) -> (w1024:bool[])
              n591 = for {
                tunnel: w1024 -> [w1083] mode=indexing
                tunnel: [w1080] -> w1050 mode=indexing
                n592 = Select(t="NG", s=w1083, f="OK") -> (s? t:f=w1080:string)
              }
              n593 = Or Array Elements(Boolean array=w1024) -> (logical OR=w1048:bool)
              n594 = for {
                tunnel: [w1055] -> w1051 mode=indexing
                tunnel: w1009 -> [w1054] mode=indexing
                tunnel: i16[] [0, 0, 1, 1, 1, 1, 1] -> [w1053] mode=indexing
                n595 = Number To Fractional String(number=w1054, precision (6)=w1053) -> (F-format string=w1055:string)  [unwired: 2 in]
              }
              n596 = case shown="True" w1048 {
                tunnel: w1024 -> [_ w1071]
                frame False {
                }
                frame True {
                  n597 = call "sub_shutdown.vi"("type"=shutdown-type."all") -> ()  [unwired: 10 in, 1 out]
                  n598 = for {
                    tunnel: w1071 -> [w1075] mode=indexing
                    tunnel: string[] ["제어단 단선", "제어단 단락", "제어단특성변화", "출력단 단선", "출력단 단락", "출력단 특성변화", "온도"] -> [w1074]
                    i -> [w1073]
                    n599 = case shown="True" w1075 {
                      tunnel: w1074 -> [_ w1078]
                      tunnel: w1073 -> [_ w1077]
                      frame False {
                      }
                      frame True {
                        n600 = Index Array(array=w1078, index=w1077) -> (element=w1076:string)
                        n601 = call "sub_log_basic.vi"("desc"=w1076, "Title"="Shutdown ") -> ()  [unwired: 9 in, 1 out]
                      }
                    }
                  }
                }
              }
              n602 = Build Array (concatenate)(w1051, w1050) -> (w1026:string[])
              n603 = call "fgv_error_rc.vi"("cmd"=init-r-w."read") -> ("Error 2"=w1034:T16)  [unwired: 10 in]
              n604 = Unbundle By Name(w1034) -> ("제어단 단락"=w1031:bool, "출력단 단락"=w1030:bool)
              n605 = Array Size(array=w1026) -> (size(s)=w1032:i32)
              n606 = Initialize Array("-", w1032) -> (w1028:string[])
              n607 = Or(x=w1031, y=w1030) -> (x .or. y?=w1029:bool)
              n608 = Select(t=w1028, s=w1029, f=w1026) -> (s? t:f=w1027:string[])
              n609 = case shown="True" w1029 {
                tunnel: [w1056 w1067] -> w1025
                tunnel: w1027 -> [w1056 w1069]
                tunnel: w1031 -> [_ w1065]
                tunnel: w1030 -> [_ w1057]
                frame False {
                }
                frame True {
                  n610 = Select(t="NG", s=w1065, f="OK") -> (s? t:f=w1062:string)
                  n611 = Replace Array Subset(array=w1069, new element=w1062, index=9) -> (w1068:string[])
                  n612 = Select(t="NG", s=w1057, f="OK") -> (s? t:f=w1058:string)
                  n613 = Replace Array Subset(array=w1068, new element=w1058, index=12) -> (w1067:string[])
                }
              }
              n614 = call "TableCnt.vi"("cnt"=cmd_tablecnt."Write", "appended array"=w1025) -> ()  [unwired: 8 in, 2 out]
            }
            frame #7 {
              # "저장"
              n615 = call "TableCnt.vi"("cnt"=cmd_tablecnt."Default") -> ("Item Names"=w1085:string[][])  [unwired: 9 in, 1 out]
              n616 = Index Array(array=w1085, index (col)=w1084) -> ()  [unwired: 1 in, 1 out]
            }
          }
        }
        frame "Oper_LV" {
          n617 = call "fgv_judgement.vi"("cmd"=rw."read") -> ("Test Judgement 2"=w1090:T20)  [unwired: 9 in, 1 out]
          n618 = call "fgv_measure_reg.vi"("cmd"=rw."read") -> ("measure_reg 2"=w1087:T21)  [unwired: 10 in]
          n619 = stacked-sequence {
            seq-local: [_ _ _ _ _ w1215 _ _] -> [_ _ _ _ _ _ w1270 _]
            seq-local: [w1100 _ _ _ _ _ _ _] -> [_ _ _ _ _ w1199 _ _]
            seq-local: [_ _ _ _ _ w1195 _ _] -> [_ _ _ _ _ _ w1229 _]
            tunnel: w1099 -> [w1112 _ _ _ _ _ _ _]
            tunnel: w1098 -> [w1111 _ _ _ _ _ _ _]
            tunnel: w1097 -> [_ w1130 _ _ _ _ _ _]
            tunnel: w1096 -> [_ _ w1145 _ _ _ _ _]
            tunnel: w1095 -> [_ _ w1144 _ _ _ _ _]
            tunnel: w1094 -> [_ _ _ w1164 _ _ _ _]
            tunnel: w1093 -> [_ _ _ _ w1183 _ _ _]
            tunnel: w1092 -> [_ _ _ _ _ w1222 _ _]
            tunnel: w1090 -> [_ _ _ _ _ w1221 _ _]
            tunnel: w1089 -> [_ _ _ _ _ _ w1234 w1302]
            tunnel: w1087 -> [w1106 w1125 w1143 w1163 w1182 w1220 w1266 _]
            frame #0 {
              n620 = Unbundle By Name(w1106) -> ("입력전류 RMS"=w1103:dbl)
              n621 = In Range and Coerce(upper limit=w1112, x=w1103, lower limit=w1111) -> (In Range?=w1100:bool)  [unwired: 1 out]
              n622 = Not(x=w1100) -> (.not. x?=w1102:bool)
              n623 = Not A Number/Path/Refnum?(number/path/refnum=w1103) -> (NaN/Path/Refnum?=w1105:bool)
              n624 = Select(t=TRUE, s=w1105, f=w1102) -> (s? t:f=w1101:bool)
              n625 = case shown="True" w1101 {
                tunnel: w1103 -> [_ w1117]
                frame False {
                }
                frame True {
                  n626 = Number To Fractional String(number=w1117) -> (F-format string=w1118:string)  [unwired: 3 in]
                  n627 = call "sub_log_basic.vi"("desc"=w1118, "Title"="### DL950 input curr spec out ") -> ()  [unwired: 9 in, 1 out]
                }
              }
              n628 = case shown="True" w1101 {
                tunnel: w1103 -> [_ w1113]
                frame False {
                }
                frame True {
                  n629 = Number To Fractional String(number=w1113) -> (F-format string=w1114:string)  [unwired: 3 in]
                  n630 = call "fgv_status-display.vi"("Mode"=system-status."Update", "detail"=w1114, "title"="Input RMS") -> ()  [unwired: 8 in, 1 out]
                }
              }
              n631 = call "fgv_error_rc.vi"("cmd"=init-r-w."read") -> ("Error 2"=w1110:T16)  [unwired: 10 in]
              n632 = Bundle By Name(cluster=w1110, "제어단 특성변화"=w1101) -> (w1109:T16)
              n633 = call "fgv_error_rc.vi"("cmd"=init-r-w."write", "Error"=w1109) -> ()  [unwired: 9 in, 1 out]
            }
            frame #1 {
              n634 = Unbundle By Name(w1125) -> ("입력전류 RMS"=w1122:dbl)
              n635 = Less Or Equal?(x=w1122, y=w1130) -> (x <= y?=w1121:bool)
              n636 = Not A Number/Path/Refnum?(number/path/refnum=w1122) -> (NaN/Path/Refnum?=w1124:bool)
              n637 = Select(t=TRUE, s=w1124, f=w1121) -> (s? t:f=w1120:bool)
              n638 = call "fgv_error_rc.vi"("cmd"=init-r-w."read") -> ("Error 2"=w1128:T16)  [unwired: 10 in]
              n639 = Bundle By Name(cluster=w1128, "제어단 단선"=w1120) -> (w1129:T16)
              n640 = case shown="True" w1120 {
                tunnel: w1130 -> [_ w1135]
                frame False {
                }
                frame True {
                  n641 = Number To Fractional String(number=w1135) -> (F-format string=w1136:string)  [unwired: 3 in]
                  n642 = call "sub_log_basic.vi"("desc"=w1136, "Title"="### DL950 input open") -> ()  [unwired: 9 in, 1 out]
                }
              }
              n643 = case shown="True" w1120 {
                tunnel: w1122 -> [_ w1131]
                frame False {
                }
                frame True {
                  n644 = Number To Fractional String(number=w1131) -> (F-format string=w1132:string)  [unwired: 3 in]
                  n645 = call "fgv_status-display.vi"("Mode"=system-status."Update", "detail"=w1132, "title"="Input RMS") -> ()  [unwired: 8 in, 1 out]
                }
              }
              n646 = call "fgv_error_rc.vi"("cmd"=init-r-w."write", "Error"=w1129) -> ()  [unwired: 9 in, 1 out]
            }
            frame #2 {
              n647 = Unbundle By Name(w1143) -> ("출력전류 RMS"=w1140:dbl)
              n648 = In Range and Coerce(upper limit=w1145, x=w1140, lower limit=w1144) -> (In Range?=w1150:bool)  [unwired: 1 out]
              n649 = Not(x=w1150) -> (.not. x?=w1139:bool)
              n650 = Not A Number/Path/Refnum?(number/path/refnum=w1140) -> (NaN/Path/Refnum?=w1142:bool)
              n651 = Select(t=TRUE, s=w1142, f=w1139) -> (s? t:f=w1138:bool)
              n652 = case shown="True" w1138 {
                tunnel: w1140 -> [_ w1155]
                frame False {
                }
                frame True {
                  n653 = Number To Fractional String(number=w1155) -> (F-format string=w1156:string)  [unwired: 3 in]
                  n654 = call "sub_log_basic.vi"("desc"=w1156, "Title"="### DL950 output curr spec out ") -> ()  [unwired: 9 in, 1 out]
                }
              }
              n655 = case shown="True" w1138 {
                tunnel: w1140 -> [_ w1151]
                frame False {
                }
                frame True {
                  n656 = Number To Fractional String(number=w1151) -> (F-format string=w1152:string)  [unwired: 3 in]
                  n657 = call "fgv_status-display.vi"("Mode"=system-status."Update", "detail"=w1152, "title"="Output RMS") -> ()  [unwired: 8 in, 1 out]
                }
              }
              n658 = call "fgv_error_rc.vi"("cmd"=init-r-w."read") -> ("Error 2"=w1149:T16)  [unwired: 10 in]
              n659 = Bundle By Name(cluster=w1149, "출력단 특성변화"=w1138) -> (w1148:T16)
              n660 = call "fgv_error_rc.vi"("cmd"=init-r-w."write", "Error"=w1148) -> ()  [unwired: 9 in, 1 out]
            }
            frame #3 {
              n661 = Unbundle By Name(w1163) -> ("출력전류 RMS"=w1159:dbl)
              n662 = Less Or Equal?(x=w1159, y=w1164) -> (x <= y?=w1160:bool)
              n663 = Not A Number/Path/Refnum?(number/path/refnum=w1159) -> (NaN/Path/Refnum?=w1162:bool)
              n664 = Select(t=TRUE, s=w1162, f=w1160) -> (s? t:f=w1158:bool)
              n665 = case shown="True" w1158 {
                tunnel: w1164 -> [_ w1173]
                frame False {
                }
                frame True {
                  n666 = Number To Fractional String(number=w1173) -> (F-format string=w1174:string)  [unwired: 3 in]
                  n667 = call "sub_log_basic.vi"("desc"=w1174, "Title"="### DL950 output open") -> ()  [unwired: 9 in, 1 out]
                }
              }
              n668 = case shown="True" w1158 {
                tunnel: w1159 -> [_ w1169]
                frame False {
                }
                frame True {
                  n669 = Number To Fractional String(number=w1169) -> (F-format string=w1170:string)  [unwired: 3 in]
                  n670 = call "fgv_status-display.vi"("Mode"=system-status."Update", "detail"=w1170, "title"="Output RMS") -> ()  [unwired: 8 in, 1 out]
                }
              }
              n671 = call "fgv_error_rc.vi"("cmd"=init-r-w."read") -> ("Error 2"=w1167:T16)  [unwired: 10 in]
              n672 = Bundle By Name(cluster=w1167, "출력단 단선"=w1158) -> (w1168:T16)
              n673 = call "fgv_error_rc.vi"("cmd"=init-r-w."write", "Error"=w1168) -> ()  [unwired: 9 in, 1 out]
            }
            frame #4 {
              n674 = Unbundle By Name(w1182) -> ("온도"=w1179:dbl)
              n675 = Less Or Equal?(x=w1179, y=w1183) -> (x <= y?=w1178:bool)
              n676 = Not(x=w1178) -> (.not. x?=w1177:bool)
              n677 = Not A Number/Path/Refnum?(number/path/refnum=w1179) -> (NaN/Path/Refnum?=w1181:bool)
              n678 = Select(t=TRUE, s=w1181, f=w1177) -> (s? t:f=w1176:bool)
              n679 = case shown="True" w1176 {
                tunnel: w1183 -> [_ w1192]
                frame False {
                }
                frame True {
                  n680 = Number To Fractional String(number=w1192) -> (F-format string=w1193:string)  [unwired: 3 in]
                  n681 = call "sub_log_basic.vi"("desc"=w1193, "Title"="### DL950 output open") -> ()  [unwired: 9 in, 1 out]
                }
              }
              n682 = case shown="True" w1176 {
                tunnel: w1179 -> [_ w1188]
                frame False {
                }
                frame True {
                  n683 = Number To Fractional String(number=w1188) -> (F-format string=w1189:string)  [unwired: 3 in]
                  n684 = call "fgv_status-display.vi"("Mode"=system-status."Update", "detail"=w1189, "title"="온도") -> ()  [unwired: 8 in, 1 out]
                }
              }
              n685 = call "fgv_error_rc.vi"("cmd"=init-r-w."read") -> ("Error 2"=w1186:T16)  [unwired: 10 in]
              n686 = Bundle By Name(cluster=w1186, "온도"=w1176) -> (w1187:T16)
              n687 = call "fgv_error_rc.vi"("cmd"=init-r-w."write", "Error"=w1187) -> ()  [unwired: 9 in, 1 out]
            }
            frame #5 {
              n688 = Unbundle By Name(w1221) -> ("출력전류 Irms[mA] Max"=w1201:dbl, "출력전류 Irms[mA] Min"=w1200:dbl)
              n689 = Unbundle By Name(w1220) -> ("입력카운트"=w1211:dbl, "출력카운트"=w1207:dbl, "출력전류 RMS"=w1204:dbl)  [unwired: 1 out]
              n690 = To Double Precision Float(number=w1222) -> ()  [unwired: 1 out]
              n691 = In Range and Coerce(upper limit=w1201, x=w1204, lower limit=w1200) -> (In Range?=w1198:bool)  [unwired: 1 out]
              n692 = Equal?(x=w1211, y=w1207) -> (x = y?=w1196:bool)
              n693 = And(x=w1199, y=w1198) -> (x .and. y?=w1197:bool)
              n694 = Or(x=w1197, y=w1196) -> (x .or. y?=w1195:bool)
              n695 = Build Array(w1195, w1198) -> (w1215:bool[])
              n696 = Number To Fractional String(number=w1204) -> (F-format string=w1203:string)  [unwired: 3 in]
              n697 = call "sub_log_basic.vi"("desc"=w1203, "Title"="출력전류") -> ("error out"=w1202:errorcluster)  [unwired: 9 in]
              n698 = Number To Decimal String(number=w1211) -> (decimal integer string=w1210:string)  [unwired: 1 in]
              n699 = call "sub_log_basic.vi"("error in"=w1202, "desc"=w1210, "Title"="입력 카운트") -> ("error out"=w1206:errorcluster)  [unwired: 8 in]
              n700 = Number To Decimal String(number=w1207) -> (decimal integer string=w1209:string)  [unwired: 1 in]
              n701 = call "sub_log_basic.vi"("error in"=w1206, "desc"=w1209, "Title"="출력 카운트") -> ()  [unwired: 8 in, 1 out]
              n702 = Not(x=w1215) -> (.not. x?=w1213:bool[])
              n703 = Array To Cluster(array=w1213) -> (cluster=w1214:cluster{"[0]":bool, "[1]":bool})
              n704 = call "fgv_curr-test-info.vi"("cmd"=rw."read") -> ("현재테스트 정보 2"=w1217:T4)  [unwired: 10 in]
              n705 = Bundle By Name(cluster=w1217, "NG"=w1214) -> (w1216:T4)
              n706 = call "fgv_curr-test-info.vi"("cmd"=rw."write", "현재테스트 정보"=w1216) -> ()  [unwired: 9 in, 1 out]
            }
            frame #6 {
              # "7"
              # "7"
              # "size 2"
              # "디스플레이"
              n707 = To Long Integer(number=w1234) -> (32bit integer=w1233:i32)
              n708 = Cluster To Array(cluster=w1266) -> (array=w1227:dbl[])
              n709 = Index Array(array=w1227) -> (element #1=w1226:dbl, element #2=w1225:dbl)  [unwired: 2 in]
              n710 = call "fgv_error_rc.vi"("cmd"=init-r-w."read") -> ("Error 2"=w1257:T16)  [unwired: 10 in]
              n711 = Build Array(w1226, w1225) -> (w1224:dbl[])
              n712 = Unbundle By Name(w1257) -> ("제어단 단선"=w1265:bool, "제어단 단락"=w1264:bool, "제어단 특성변화"=w1263:bool, "출력단 단선"=w1262:bool, "출력단 단락"=w1261:bool, "출력단 특성변화"=w1260:bool, "온도"=w1259:bool)
              n713 = Select(t=dbl[] [1.0, 1.0] ("array"), s=w1229, f=w1224) -> (s? t:f=w1223:dbl[])
              n714 = call "count_run 1.vi"("cmd"=cmd_count."count", "CH"=w1233, "Array_Count"=w1223) -> ("Array_data"=w1241:dbl[][])  [unwired: 7 in, 1 out]
              n715 = Index Array(array=w1241, index (row)=w1233) -> (element=w1240:dbl[])  [unwired: 1 in]
              n716 = Index Array(array=w1240) -> (element #1=w1238:dbl, element #2=w1235:dbl)  [unwired: 2 in]
              n717 = Build Array(w1265, w1264, w1263, w1262, w1261, w1260, w1259) -> (w1255:bool[])
              n718 = Replace Array Subset(array=w1227, new element=w1238, index=0) -> (w1236:dbl[])
              n719 = Not(x=w1270) -> (.not. x?=w1256:bool[])
              n720 = Replace Array Subset(array=w1236, new element=w1235, index=1) -> (w1231:dbl[])
              n721 = Build Array (concatenate)(w1256, w1255) -> (w1243:bool[])
              n722 = Or Array Elements(Boolean array=w1243) -> (logical OR=w1267:bool)
              n723 = for {
                tunnel: w1243 -> [w1301] mode=indexing
                tunnel: [w1298] -> w1269 mode=indexing
                n724 = Select(t="NG", s=w1301, f="OK") -> (s? t:f=w1298:string)
              }
              n725 = case shown="True" w1267 {
                tunnel: w1243 -> [_ w1289]
                frame False {
                }
                frame True {
                  n726 = call "sub_shutdown.vi"("type"=shutdown-type."all") -> ()  [unwired: 10 in, 1 out]
                  n727 = for {
                    tunnel: w1289 -> [w1293] mode=indexing
                    tunnel: string[] ["제어단 단선", "제어단 단락", "제어단특성변화", "출력단 단선", "출력단 단락", "출력단 특성변화", "온도"] -> [w1292]
                    i -> [w1291]
                    n728 = case shown="True" w1293 {
                      tunnel: w1292 -> [_ w1296]
                      tunnel: w1291 -> [_ w1295]
                      frame False {
                      }
                      frame True {
                        n729 = Index Array(array=w1296, index=w1295) -> (element=w1294:string)
                        n730 = call "sub_log_basic.vi"("desc"=w1294, "Title"="Shutdown ") -> ()  [unwired: 9 in, 1 out]
                      }
                    }
                  }
                }
              }
              n731 = for {
                tunnel: [w1273] -> w1230 mode=indexing
                tunnel: w1231 -> [w1272] mode=indexing
                tunnel: i16[] [0, 0, 1, 1, 1, 1, 1] -> [w1271] mode=indexing
                n732 = Number To Fractional String(number=w1272, precision (6)=w1271) -> (F-format string=w1273:string)  [unwired: 2 in]
              }
              n733 = Build Array (concatenate)(w1230, w1269) -> (w1245:string[])
              n734 = call "fgv_error_rc.vi"("cmd"=init-r-w."read") -> ("Error 2"=w1253:T16)  [unwired: 10 in]
              n735 = Unbundle By Name(w1253) -> ("제어단 단락"=w1250:bool, "출력단 단락"=w1249:bool)
              n736 = Array Size(array=w1245) -> (size(s)=w1251:i32)
              n737 = Initialize Array("-", w1251) -> (w1247:string[])
              n738 = Or(x=w1250, y=w1249) -> (x .or. y?=w1248:bool)
              n739 = Select(t=w1247, s=w1248, f=w1245) -> (s? t:f=w1246:string[])
              n740 = case shown="True" w1248 {
                tunnel: [w1274 w1285] -> w1244
                tunnel: w1246 -> [w1274 w1287]
                tunnel: w1250 -> [_ w1283]
                tunnel: w1249 -> [_ w1275]
                frame False {
                }
                frame True {
                  n741 = Select(t="NG", s=w1283, f="OK") -> (s? t:f=w1280:string)
                  n742 = Replace Array Subset(array=w1287, new element=w1280, index=10) -> (w1286:string[])
                  n743 = Select(t="NG", s=w1275, f="OK") -> (s? t:f=w1276:string)
                  n744 = Replace Array Subset(array=w1286, new element=w1276, index=13) -> (w1285:string[])
                }
              }
              n745 = call "TableCnt.vi"("cnt"=cmd_tablecnt."Write", "appended array"=w1244) -> ()  [unwired: 8 in, 2 out]
            }
            frame #7 {
              # "저장"
              n746 = call "TableCnt.vi"("cnt"=cmd_tablecnt."Default") -> ("Item Names"=w1303:string[][])  [unwired: 9 in, 1 out]
              n747 = Index Array(array=w1303, index (col)=w1302) -> ()  [unwired: 1 in, 1 out]
            }
          }
        }
        frame "ContR_LV" {
          n748 = call "fgv_measure_ContR.vi"("cmd"=rw."read") -> ("measure_ContR Out"=w1305:T23)  [unwired: 9 in, 1 out]
          n749 = call "fgv_judgement.vi"("cmd"=rw."read") -> ("Test Judgement 2"=w1308:T20)  [unwired: 9 in, 1 out]
          n750 = stacked-sequence {
            seq-local: [_ _ _ _ _ w1434 _ _] -> [_ _ _ _ _ _ w1489 _]
            seq-local: [w1318 _ _ _ _ _ _ _] -> [_ _ _ _ _ w1417 _ _]
            seq-local: [_ _ _ _ _ w1413 _ _] -> [_ _ _ _ _ _ w1444 _]
            tunnel: w1317 -> [w1330 _ _ _ _ _ _ _]
            tunnel: w1316 -> [w1329 _ _ _ _ _ _ _]
            tunnel: w1315 -> [_ w1348 _ _ _ _ _ _]
            tunnel: w1314 -> [_ _ w1363 _ _ _ _ _]
            tunnel: w1313 -> [_ _ w1362 _ _ _ _ _]
            tunnel: w1312 -> [_ _ _ w1382 _ _ _ _]
            tunnel: w1311 -> [_ _ _ _ w1401 _ _ _]
            tunnel: w1310 -> [_ _ _ _ _ w1441 _ _]
            tunnel: w1308 -> [_ _ _ _ _ w1440 _ _]
            tunnel: w1307 -> [_ _ _ _ _ _ w1450 w1521]
            tunnel: w1305 -> [w1324 w1343 w1361 w1381 w1400 w1439 w1485 _]
            frame #0 {
              n751 = Unbundle By Name(w1324) -> ("입력전류 RMS"=w1321:dbl)
              n752 = In Range and Coerce(upper limit=w1330, x=w1321, lower limit=w1329) -> (In Range?=w1318:bool)  [unwired: 1 out]
              n753 = Not(x=w1318) -> (.not. x?=w1320:bool)
              n754 = Not A Number/Path/Refnum?(number/path/refnum=w1321) -> (NaN/Path/Refnum?=w1323:bool)
              n755 = Select(t=TRUE, s=w1323, f=w1320) -> (s? t:f=w1319:bool)
              n756 = case shown="True" w1319 {
                tunnel: w1321 -> [_ w1335]
                frame False {
                }
                frame True {
                  n757 = Number To Fractional String(number=w1335) -> (F-format string=w1336:string)  [unwired: 3 in]
                  n758 = call "sub_log_basic.vi"("desc"=w1336, "Title"="### DL950 input curr spec out ") -> ()  [unwired: 9 in, 1 out]
                }
              }
              n759 = case shown="True" w1319 {
                tunnel: w1321 -> [_ w1331]
                frame False {
                }
                frame True {
                  n760 = Number To Fractional String(number=w1331) -> (F-format string=w1332:string)  [unwired: 3 in]
                  n761 = call "fgv_status-display.vi"("Mode"=system-status."Update", "detail"=w1332, "title"="Input RMS") -> ()  [unwired: 8 in, 1 out]
                }
              }
              n762 = call "fgv_error_rc.vi"("cmd"=init-r-w."read") -> ("Error 2"=w1328:T16)  [unwired: 10 in]
              n763 = Bundle By Name(cluster=w1328, "제어단 특성변화"=w1319) -> (w1327:T16)
              n764 = call "fgv_error_rc.vi"("cmd"=init-r-w."write", "Error"=w1327) -> ()  [unwired: 9 in, 1 out]
            }
            frame #1 {
              n765 = Unbundle By Name(w1343) -> ("입력전류 RMS"=w1340:dbl)
              n766 = Less Or Equal?(x=w1340, y=w1348) -> (x <= y?=w1339:bool)
              n767 = Not A Number/Path/Refnum?(number/path/refnum=w1340) -> (NaN/Path/Refnum?=w1342:bool)
              n768 = Select(t=TRUE, s=w1342, f=w1339) -> (s? t:f=w1338:bool)
              n769 = call "fgv_error_rc.vi"("cmd"=init-r-w."read") -> ("Error 2"=w1346:T16)  [unwired: 10 in]
              n770 = Bundle By Name(cluster=w1346, "제어단 단선"=w1338) -> (w1347:T16)
              n771 = case shown="True" w1338 {
                tunnel: w1348 -> [_ w1353]
                frame False {
                }
                frame True {
                  n772 = Number To Fractional String(number=w1353) -> (F-format string=w1354:string)  [unwired: 3 in]
                  n773 = call "sub_log_basic.vi"("desc"=w1354, "Title"="### DL950 input open") -> ()  [unwired: 9 in, 1 out]
                }
              }
              n774 = case shown="True" w1338 {
                tunnel: w1340 -> [_ w1349]
                frame False {
                }
                frame True {
                  n775 = Number To Fractional String(number=w1349) -> (F-format string=w1350:string)  [unwired: 3 in]
                  n776 = call "fgv_status-display.vi"("Mode"=system-status."Update", "detail"=w1350, "title"="Input RMS") -> ()  [unwired: 8 in, 1 out]
                }
              }
              n777 = call "fgv_error_rc.vi"("cmd"=init-r-w."write", "Error"=w1347) -> ()  [unwired: 9 in, 1 out]
            }
            frame #2 {
              n778 = Unbundle By Name(w1361) -> ("출력전류 RMS"=w1358:dbl)
              n779 = In Range and Coerce(upper limit=w1363, x=w1358, lower limit=w1362) -> (In Range?=w1368:bool)  [unwired: 1 out]
              n780 = Not(x=w1368) -> (.not. x?=w1357:bool)
              n781 = Not A Number/Path/Refnum?(number/path/refnum=w1358) -> (NaN/Path/Refnum?=w1360:bool)
              n782 = Select(t=TRUE, s=w1360, f=w1357) -> (s? t:f=w1356:bool)
              n783 = case shown="True" w1356 {
                tunnel: w1358 -> [_ w1373]
                frame False {
                }
                frame True {
                  n784 = Number To Fractional String(number=w1373) -> (F-format string=w1374:string)  [unwired: 3 in]
                  n785 = call "sub_log_basic.vi"("desc"=w1374, "Title"="### DL950 output curr spec out ") -> ()  [unwired: 9 in, 1 out]
                }
              }
              n786 = case shown="True" w1356 {
                tunnel: w1358 -> [_ w1369]
                frame False {
                }
                frame True {
                  n787 = Number To Fractional String(number=w1369) -> (F-format string=w1370:string)  [unwired: 3 in]
                  n788 = call "fgv_status-display.vi"("Mode"=system-status."Update", "detail"=w1370, "title"="Output RMS") -> ()  [unwired: 8 in, 1 out]
                }
              }
              n789 = call "fgv_error_rc.vi"("cmd"=init-r-w."read") -> ("Error 2"=w1367:T16)  [unwired: 10 in]
              n790 = Bundle By Name(cluster=w1367, "출력단 특성변화"=w1356) -> (w1366:T16)
              n791 = call "fgv_error_rc.vi"("cmd"=init-r-w."write", "Error"=w1366) -> ()  [unwired: 9 in, 1 out]
            }
            frame #3 {
              n792 = Unbundle By Name(w1381) -> ("출력전류 RMS"=w1377:dbl)
              n793 = Less Or Equal?(x=w1377, y=w1382) -> (x <= y?=w1378:bool)
              n794 = Not A Number/Path/Refnum?(number/path/refnum=w1377) -> (NaN/Path/Refnum?=w1380:bool)
              n795 = Select(t=TRUE, s=w1380, f=w1378) -> (s? t:f=w1376:bool)
              n796 = case shown="True" w1376 {
                tunnel: w1382 -> [_ w1391]
                frame False {
                }
                frame True {
                  n797 = Number To Fractional String(number=w1391) -> (F-format string=w1392:string)  [unwired: 3 in]
                  n798 = call "sub_log_basic.vi"("desc"=w1392, "Title"="### DL950 output open") -> ()  [unwired: 9 in, 1 out]
                }
              }
              n799 = case shown="True" w1376 {
                tunnel: w1377 -> [_ w1387]
                frame False {
                }
                frame True {
                  n800 = Number To Fractional String(number=w1387) -> (F-format string=w1388:string)  [unwired: 3 in]
                  n801 = call "fgv_status-display.vi"("Mode"=system-status."Update", "detail"=w1388, "title"="Output RMS") -> ()  [unwired: 8 in, 1 out]
                }
              }
              n802 = call "fgv_error_rc.vi"("cmd"=init-r-w."read") -> ("Error 2"=w1385:T16)  [unwired: 10 in]
              n803 = Bundle By Name(cluster=w1385, "출력단 단선"=w1376) -> (w1386:T16)
              n804 = call "fgv_error_rc.vi"("cmd"=init-r-w."write", "Error"=w1386) -> ()  [unwired: 9 in, 1 out]
            }
            frame #4 {
              n805 = Unbundle By Name(w1400) -> ("온도"=w1397:dbl)
              n806 = Less Or Equal?(x=w1397, y=w1401) -> (x <= y?=w1396:bool)
              n807 = Not(x=w1396) -> (.not. x?=w1395:bool)
              n808 = Not A Number/Path/Refnum?(number/path/refnum=w1397) -> (NaN/Path/Refnum?=w1399:bool)
              n809 = Select(t=TRUE, s=w1399, f=w1395) -> (s? t:f=w1394:bool)
              n810 = case shown="True" w1394 {
                tunnel: w1401 -> [_ w1410]
                frame False {
                }
                frame True {
                  n811 = Number To Fractional String(number=w1410) -> (F-format string=w1411:string)  [unwired: 3 in]
                  n812 = call "sub_log_basic.vi"("desc"=w1411, "Title"="### DL950 output open") -> ()  [unwired: 9 in, 1 out]
                }
              }
              n813 = case shown="True" w1394 {
                tunnel: w1397 -> [_ w1406]
                frame False {
                }
                frame True {
                  n814 = Number To Fractional String(number=w1406) -> (F-format string=w1407:string)  [unwired: 3 in]
                  n815 = call "fgv_status-display.vi"("Mode"=system-status."Update", "detail"=w1407, "title"="온도") -> ()  [unwired: 8 in, 1 out]
                }
              }
              n816 = call "fgv_error_rc.vi"("cmd"=init-r-w."read") -> ("Error 2"=w1404:T16)  [unwired: 10 in]
              n817 = Bundle By Name(cluster=w1404, "온도"=w1394) -> (w1405:T16)
              n818 = call "fgv_error_rc.vi"("cmd"=init-r-w."write", "Error"=w1405) -> ()  [unwired: 9 in, 1 out]
            }
            frame #5 {
              n819 = Unbundle By Name(w1440) -> ("접촉저항[mOhm] Max"=w1418:dbl, "접촉저항[mOhm] Min"=w1419:dbl)  [unwired: 2 out]
              n820 = Unbundle By Name(w1439) -> ("입력카운트"=w1430:dbl, "출력카운트"=w1426:dbl, "출력전류 RMS"=w1423:dbl, "접촉저항"=w1420:dbl)
              n821 = To Double Precision Float(number=w1441) -> ()  [unwired: 1 out]
              n822 = Equal?(x=w1430, y=w1426) -> (x = y?=w1414:bool)
              n823 = In Range and Coerce(upper limit=w1418, x=w1420, lower limit=w1419) -> (In Range?=w1416:bool)  [unwired: 1 out]
              n824 = And(x=w1417, y=w1416) -> (x .and. y?=w1415:bool)
              n825 = Or(x=w1415, y=w1414) -> (x .or. y?=w1413:bool)
              n826 = Number To Fractional String(number=w1423) -> (F-format string=w1422:string)  [unwired: 3 in]
              n827 = Build Array(w1413, w1416) -> (w1434:bool[])
              n828 = call "sub_log_basic.vi"("desc"=w1422, "Title"="출력전류") -> ("error out"=w1421:errorcluster)  [unwired: 9 in]
              n829 = Number To Decimal String(number=w1430) -> (decimal integer string=w1429:string)  [unwired: 1 in]
              n830 = call "sub_log_basic.vi"("error in"=w1421, "desc"=w1429, "Title"="입력 카운트") -> ("error out"=w1425:errorcluster)  [unwired: 8 in]
              n831 = Number To Decimal String(number=w1426) -> (decimal integer string=w1428:string)  [unwired: 1 in]
              n832 = call "sub_log_basic.vi"("error in"=w1425, "desc"=w1428, "Title"="출력 카운트") -> ()  [unwired: 8 in, 1 out]
              n833 = Not(x=w1434) -> (.not. x?=w1432:bool[])
              n834 = Array To Cluster(array=w1432) -> (cluster=w1433:cluster{"[0]":bool, "[1]":bool})
              n835 = call "fgv_curr-test-info.vi"("cmd"=rw."read") -> ("현재테스트 정보 2"=w1436:T4)  [unwired: 10 in]
              n836 = Bundle By Name(cluster=w1436, "NG"=w1433) -> (w1435:T4)
              n837 = call "fgv_curr-test-info.vi"("cmd"=rw."write", "현재테스트 정보"=w1435) -> ()  [unwired: 9 in, 1 out]
            }
            frame #6 {
              # "7"
              # "10"
              # "2"
              # "디스플레이"
              n838 = To Long Integer(number=w1450) -> (32bit integer=w1449:i32)
              n839 = Cluster To Array(cluster=w1485) -> (array=w1451:dbl[])
              n840 = Index Array(array=w1451) -> (element #1=w1458:dbl, element #2=w1457:dbl)  [unwired: 2 in]
              n841 = Build Array(w1458, w1457) -> (w1443:dbl[])
              n842 = call "fgv_error_rc.vi"("cmd"=init-r-w."read") -> ("Error 2"=w1476:T16)  [unwired: 10 in]
              n843 = Select(t=dbl[] [1.0, 1.0] ("array"), s=w1444, f=w1443) -> (s? t:f=w1442:dbl[])
              n844 = Unbundle By Name(w1476) -> ("제어단 단선"=w1484:bool, "제어단 단락"=w1483:bool, "제어단 특성변화"=w1482:bool, "출력단 단선"=w1481:bool, "출력단 단락"=w1480:bool, "출력단 특성변화"=w1479:bool, "온도"=w1478:bool)
              n845 = call "count_run 1.vi"("cmd"=cmd_count."count", "CH"=w1449, "Array_Count"=w1442) -> ("Array_data"=w1460:dbl[][])  [unwired: 7 in, 1 out]
              n846 = Index Array(array=w1460, index (row)=w1449) -> (element=w1459:dbl[])  [unwired: 1 in]
              n847 = Index Array(array=w1459) -> (element #1=w1455:dbl, element #2=w1452:dbl)  [unwired: 2 in]
              n848 = Replace Array Subset(array=w1451, new element=w1455, index=0) -> (w1453:dbl[])
              n849 = Build Array(w1484, w1483, w1482, w1481, w1480, w1479, w1478) -> (w1474:bool[])
              n850 = Not(x=w1489) -> (.not. x?=w1475:bool[])
              n851 = Replace Array Subset(array=w1453, new element=w1452, index=1) -> (w1447:dbl[])
              n852 = Build Array (concatenate)(w1475, w1474) -> (w1462:bool[])
              n853 = Or Array Elements(Boolean array=w1462) -> (logical OR=w1486:bool)
              n854 = for {
                tunnel: w1462 -> [w1520] mode=indexing
                tunnel: [w1517] -> w1488 mode=indexing
                n855 = Select(t="NG", s=w1520, f="OK") -> (s? t:f=w1517:string)
              }
              n856 = case shown="True" w1486 {
                tunnel: w1462 -> [_ w1508]
                frame False {
                }
                frame True {
                  n857 = call "sub_shutdown.vi"("type"=shutdown-type."all") -> ()  [unwired: 10 in, 1 out]
                  n858 = for {
                    tunnel: w1508 -> [w1512] mode=indexing
                    tunnel: string[] ["제어단 단선", "제어단 단락", "제어단특성변화", "출력단 단선", "출력단 단락", "출력단 특성변화", "온도"] -> [w1511]
                    i -> [w1510]
                    n859 = case shown="True" w1512 {
                      tunnel: w1511 -> [_ w1515]
                      tunnel: w1510 -> [_ w1514]
                      frame False {
                      }
                      frame True {
                        n860 = Index Array(array=w1515, index=w1514) -> (element=w1513:string)
                        n861 = call "sub_log_basic.vi"("desc"=w1513, "Title"="Shutdown ") -> ()  [unwired: 9 in, 1 out]
                      }
                    }
                  }
                }
              }
              n862 = for {
                tunnel: [w1492] -> w1446 mode=indexing
                tunnel: w1447 -> [w1491] mode=indexing
                tunnel: i16[] [0, 0, 1, 1, 1, 1, 3, 1, 1, 1] -> [w1490] mode=indexing
                n863 = Number To Fractional String(number=w1491, precision (6)=w1490) -> (F-format string=w1492:string)  [unwired: 2 in]
              }
              n864 = Build Array (concatenate)(w1446, w1488) -> (w1464:string[])
              n865 = call "fgv_error_rc.vi"("cmd"=init-r-w."read") -> ("Error 2"=w1472:T16)  [unwired: 10 in]
              n866 = Unbundle By Name(w1472) -> ("제어단 단락"=w1469:bool, "출력단 단락"=w1468:bool)
              n867 = Array Size(array=w1464) -> (size(s)=w1470:i32)
              n868 = Initialize Array("-", w1470) -> (w1466:string[])
              n869 = Or(x=w1469, y=w1468) -> (x .or. y?=w1467:bool)
              n870 = Select(t=w1466, s=w1467, f=w1464) -> (s? t:f=w1465:string[])
              n871 = case shown="True" w1467 {
                tunnel: [w1493 w1504] -> w1463
                tunnel: w1465 -> [w1493 w1506]
                tunnel: w1469 -> [_ w1502]
                tunnel: w1468 -> [_ w1494]
                frame False {
                }
                frame True {
                  n872 = Select(t="NG", s=w1502, f="OK") -> (s? t:f=w1499:string)
                  n873 = Replace Array Subset(array=w1506, new element=w1499, index=13) -> (w1505:string[])
                  n874 = Select(t="NG", s=w1494, f="OK") -> (s? t:f=w1495:string)
                  n875 = Replace Array Subset(array=w1505, new element=w1495, index=16) -> (w1504:string[])
                }
              }
              n876 = call "TableCnt.vi"("cnt"=cmd_tablecnt."Write", "appended array"=w1463) -> ()  [unwired: 8 in, 2 out]
            }
            frame #7 {
              # "저장"
              n877 = call "TableCnt.vi"("cnt"=cmd_tablecnt."Default") -> ("Item Names"=w1522:string[][])  [unwired: 9 in, 1 out]
              n878 = Index Array(array=w1522, index (col)=w1521) -> ()  [unwired: 1 in, 1 out]
            }
          }
        }
        frame "Oper_HV" {
          n879 = call "fgv_judgement.vi"("cmd"=rw."read") -> ("Test Judgement 2"=w1527:T20)  [unwired: 9 in, 1 out]
          n880 = call "fgv_measure_rc.vi"("cmd"=rw."read") -> ("measure_rc 2"=w1524:T22)  [unwired: 10 in]
          n881 = stacked-sequence {
            seq-local: [_ _ _ _ _ w1663 _ _] -> [_ _ _ _ _ _ w1691 _]
            seq-local: [w1537 _ _ _ _ _ _ _] -> [_ _ _ _ _ _ _ _]
            tunnel: w1536 -> [w1549 _ _ _ _ _ _ _]
            tunnel: w1535 -> [w1548 _ _ _ _ _ _ _]
            tunnel: w1534 -> [_ w1567 _ _ _ _ _ _]
            tunnel: w1533 -> [_ _ w1582 _ _ _ _ _]
            tunnel: w1532 -> [_ _ w1581 _ _ _ _ _]
            tunnel: w1531 -> [_ _ _ w1601 _ _ _ _]
            tunnel: w1530 -> [_ _ _ _ w1620 _ _ _]
            tunnel: w1529 -> [_ _ _ _ _ w1648 w1712 _]
            tunnel: w1527 -> [_ _ _ _ _ w1664 _ _]
            tunnel: w1526 -> [_ _ _ _ _ _ w1683 _]
            tunnel: w1524 -> [w1543 w1562 w1580 w1600 w1619 w1665 w1676 _]
            frame #0 {
              n882 = Unbundle By Name(w1543) -> ("입력전류 RMS"=w1542:dbl)
              n883 = In Range and Coerce(upper limit=w1549, x=w1542, lower limit=w1548) -> (In Range?=w1537:bool)  [unwired: 1 out]
              n884 = Not(x=w1537) -> (.not. x?=w1540:bool)
              n885 = Not A Number/Path/Refnum?(number/path/refnum=w1542) -> (NaN/Path/Refnum?=w1541:bool)
              n886 = Select(t=TRUE, s=w1541, f=w1540) -> (s? t:f=w1539:bool)
              n887 = case shown="True" w1539 {
                tunnel: w1542 -> [_ w1554]
                frame False {
                }
                frame True {
                  n888 = Number To Fractional String(number=w1554) -> (F-format string=w1555:string)  [unwired: 3 in]
                  n889 = call "sub_log_basic.vi"("desc"=w1555, "Title"="### DL950 input curr spec out ") -> ()  [unwired: 9 in, 1 out]
                }
              }
              n890 = case shown="True" w1539 {
                tunnel: w1542 -> [_ w1550]
                frame False {
                }
                frame True {
                  n891 = Number To Fractional String(number=w1550) -> (F-format string=w1551:string)  [unwired: 3 in]
                  n892 = call "fgv_status-display.vi"("Mode"=system-status."Update", "detail"=w1551, "title"="Input RMS") -> ()  [unwired: 8 in, 1 out]
                }
              }
              n893 = call "fgv_error_rc.vi"("cmd"=init-r-w."read") -> ("Error 2"=w1547:T16)  [unwired: 10 in]
              n894 = Bundle By Name(cluster=w1547, "제어단 특성변화"=w1539) -> (w1546:T16)
              n895 = call "fgv_error_rc.vi"("cmd"=init-r-w."write", "Error"=w1546) -> ()  [unwired: 9 in, 1 out]
            }
            frame #1 {
              n896 = Unbundle By Name(w1562) -> ("입력전류 RMS"=w1559:dbl)
              n897 = Less Or Equal?(x=w1559, y=w1567) -> (x <= y?=w1558:bool)
              n898 = Not A Number/Path/Refnum?(number/path/refnum=w1559) -> (NaN/Path/Refnum?=w1561:bool)
              n899 = Select(t=TRUE, s=w1561, f=w1558) -> (s? t:f=w1557:bool)
              n900 = case shown="True" w1557 {
                tunnel: w1559 -> [_ w1568]
                frame False {
                }
                frame True {
                  n901 = Number To Fractional String(number=w1568) -> (F-format string=w1569:string)  [unwired: 3 in]
                  n902 = call "fgv_status-display.vi"("Mode"=system-status."Update", "detail"=w1569, "title"="Input RMS") -> ()  [unwired: 8 in, 1 out]
                }
              }
              n903 = case shown="True" w1557 {
                tunnel: w1567 -> [_ w1572]
                frame False {
                }
                frame True {
                  n904 = Number To Fractional String(number=w1572) -> (F-format string=w1573:string)  [unwired: 3 in]
                  n905 = call "sub_log_basic.vi"("desc"=w1573, "Title"="### DL950 input open") -> ()  [unwired: 9 in, 1 out]
                }
              }
              n906 = call "fgv_error_rc.vi"("cmd"=init-r-w."read") -> ("Error 2"=w1565:T16)  [unwired: 10 in]
              n907 = Bundle By Name(cluster=w1565, "제어단 단선"=w1557) -> (w1566:T16)
              n908 = call "fgv_error_rc.vi"("cmd"=init-r-w."write", "Error"=w1566) -> ()  [unwired: 9 in, 1 out]
            }
            frame #2 {
              n909 = Unbundle By Name(w1580) -> ("출력전류 RMS"=w1577:dbl)
              n910 = In Range and Coerce(upper limit=w1582, x=w1577, lower limit=w1581) -> (In Range?=w1587:bool)  [unwired: 1 out]
              n911 = Not(x=w1587) -> (.not. x?=w1576:bool)
              n912 = Not A Number/Path/Refnum?(number/path/refnum=w1577) -> (NaN/Path/Refnum?=w1579:bool)
              n913 = Select(t=TRUE, s=w1579, f=w1576) -> (s? t:f=w1575:bool)
              n914 = case shown="True" w1575 {
                tunnel: w1577 -> [_ w1588]
                frame False {
                }
                frame True {
                  n915 = Number To Fractional String(number=w1588) -> (F-format string=w1589:string)  [unwired: 3 in]
                  n916 = call "fgv_status-display.vi"("Mode"=system-status."Update", "detail"=w1589, "title"="Output RMS") -> ()  [unwired: 8 in, 1 out]
                }
              }
              n917 = case shown="False" w1575 {
                tunnel: w1577 -> [_ w1592]
                frame False {
                }
                frame True {
                  n918 = Number To Fractional String(number=w1592) -> (F-format string=w1593:string)  [unwired: 3 in]
                  n919 = call "sub_log_basic.vi"("desc"=w1593, "Title"="### DL950 output curr spec out ") -> ()  [unwired: 9 in, 1 out]
                }
              }
              n920 = call "fgv_error_rc.vi"("cmd"=init-r-w."read") -> ("Error 2"=w1586:T16)  [unwired: 10 in]
              n921 = Bundle By Name(cluster=w1586, "출력단 특성변화"=w1575) -> (w1585:T16)
              n922 = call "fgv_error_rc.vi"("cmd"=init-r-w."write", "Error"=w1585) -> ()  [unwired: 9 in, 1 out]
            }
            frame #3 {
              n923 = Unbundle By Name(w1600) -> ("출력전류 RMS"=w1597:dbl)
              n924 = Less Or Equal?(x=w1597, y=w1601) -> (x <= y?=w1596:bool)
              n925 = Not A Number/Path/Refnum?(number/path/refnum=w1597) -> (NaN/Path/Refnum?=w1599:bool)
              n926 = Select(t=TRUE, s=w1599, f=w1596) -> (s? t:f=w1595:bool)
              n927 = case shown="True" w1595 {
                tunnel: w1597 -> [_ w1606]
                frame False {
                }
                frame True {
                  n928 = Number To Fractional String(number=w1606) -> (F-format string=w1607:string)  [unwired: 3 in]
                  n929 = call "fgv_status-display.vi"("Mode"=system-status."Update", "detail"=w1607, "title"="Output RMS") -> ()  [unwired: 8 in, 1 out]
                }
              }
              n930 = case shown="True" w1595 {
                tunnel: w1601 -> [_ w1610]
                frame False {
                }
                frame True {
                  n931 = Number To Fractional String(number=w1610) -> (F-format string=w1611:string)  [unwired: 3 in]
                  n932 = call "sub_log_basic.vi"("desc"=w1611, "Title"="### DL950 output open") -> ()  [unwired: 9 in, 1 out]
                }
              }
              n933 = call "fgv_error_rc.vi"("cmd"=init-r-w."read") -> ("Error 2"=w1604:T16)  [unwired: 10 in]
              n934 = Bundle By Name(cluster=w1604, "출력단 단선"=w1595) -> (w1605:T16)
              n935 = call "fgv_error_rc.vi"("cmd"=init-r-w."write", "Error"=w1605) -> ()  [unwired: 9 in, 1 out]
            }
            frame #4 {
              n936 = Unbundle By Name(w1619) -> ("온도"=w1616:dbl)
              n937 = Not A Number/Path/Refnum?(number/path/refnum=w1616) -> (NaN/Path/Refnum?=w1618:bool)
              n938 = Less Or Equal?(x=w1616, y=w1620) -> (x <= y?=w1615:bool)
              n939 = Not(x=w1615) -> (.not. x?=w1614:bool)
              n940 = Select(t=TRUE, s=w1618, f=w1614) -> (s? t:f=w1613:bool)
              n941 = case shown="True" w1613 {
                tunnel: w1620 -> [_ w1629]
                frame False {
                }
                frame True {
                  n942 = Number To Fractional String(number=w1629) -> (F-format string=w1630:string)  [unwired: 3 in]
                  n943 = call "sub_log_basic.vi"("desc"=w1630, "Title"="### DL950 output open") -> ()  [unwired: 9 in, 1 out]
                }
              }
              n944 = case shown="True" w1613 {
                tunnel: w1616 -> [_ w1625]
                frame False {
                }
                frame True {
                  n945 = Number To Fractional String(number=w1625) -> (F-format string=w1626:string)  [unwired: 3 in]
                  n946 = call "fgv_status-display.vi"("Mode"=system-status."Update", "detail"=w1626, "title"="Temp") -> ()  [unwired: 8 in, 1 out]
                }
              }
              n947 = call "fgv_error_rc.vi"("cmd"=init-r-w."read") -> ("Error 2"=w1623:T16)  [unwired: 10 in]
              n948 = Bundle By Name(cluster=w1623, "온도"=w1613) -> (w1624:T16)
              n949 = call "fgv_error_rc.vi"("cmd"=init-r-w."write", "Error"=w1624) -> ()  [unwired: 9 in, 1 out]
            }
            frame #5 {
              n950 = Unbundle By Name(w1664) -> ("전압 63%[mS] Max"=w1647:dbl, "전압 63%[mS] Min"=w1646:dbl, "전압 98%[mS] Max"=w1645:dbl, "전압 98%[mS] Min"=w1644:dbl, "전류 37%[mS] Max"=w1643:dbl, "전류 37%[mS] Min"=w1642:dbl, "출력전류 Irms[mA] Max"=w1641:dbl, "출력전류 Irms[mA] Min"=w1640:dbl, "접촉저항[mOhm] Max"=w1639:dbl, "접촉저항[mOhm] Min"=w1638:dbl)
              n951 = Unbundle By Name(w1665) -> ("입력카운트"=w1632:dbl, "Rising Time 63%"=w1662:dbl, "Rising Time 98%"=w1661:dbl, "Failing Time 37%"=w1660:dbl, "출력전류 RMS"=w1659:dbl, "접촉저항"=w1658:dbl, "방전전압"=w1635:dbl)  [unwired: 1 out]
              n952 = Number To Decimal String(number=w1648) -> (decimal integer string=w1650:string)  [unwired: 1 in]
              n953 = call "fgv_rc-config.vi"("cmd"=rw."read") -> ("Testconfig out"=w1636:T17)  [unwired: 9 in, 1 out]
              n954 = Unbundle By Name(w1636) -> ("방전 기준[V]"=w1634:dbl)
              n955 = call "sub_log_basic.vi"("desc"=w1650, "Title"="input count") -> ()  [unwired: 9 in, 1 out]
              n956 = Build Array(w1632, w1662, w1661, w1660, w1659, w1658) -> (w1657:dbl[])
              n957 = Less Or Equal?(x=w1635, y=w1634) -> (x <= y?=w1633:bool)
              n958 = In Range and Coerce(upper limit=w1647, x=w1662, lower limit=w1646) -> (In Range?=w1656:bool)  [unwired: 1 out]
              n959 = In Range and Coerce(upper limit=w1645, x=w1661, lower limit=w1644) -> (In Range?=w1655:bool)  [unwired: 1 out]
              n960 = In Range and Coerce(upper limit=w1643, x=w1660, lower limit=w1642) -> (In Range?=w1654:bool)  [unwired: 1 out]
              n961 = In Range and Coerce(upper limit=w1641, x=w1659, lower limit=w1640) -> (In Range?=w1653:bool)  [unwired: 1 out]
              n962 = In Range and Coerce(upper limit=w1639, x=w1658, lower limit=w1638) -> (In Range?=w1652:bool)  [unwired: 1 out]
              n963 = Compound Arithmetic op=AND(w1656, w1655, w1654, w1653, w1652, w1633) -> (w1651:bool)
              n964 = Build Array(w1651, w1656, w1655, w1654, w1653, w1652, w1633) -> (w1663:bool[])
              n965 = for {
                tunnel: w1663 -> [w1669] mode=indexing
                tunnel: w1657 -> [w1668] mode=indexing
                i -> [w1667]
                n966 = Not(x=w1669) -> (.not. x?=w1666:bool)
                n967 = case shown="True" w1666 {
                  tunnel: w1668 -> [_ w1674]
                  tunnel: w1667 -> [_ w1671]
                  frame False {
                  }
                  frame True {
                    n968 = Number To Fractional String(number=w1674) -> (F-format string=w1673:string)  [unwired: 3 in]
                    n969 = Index Array(array=string[] ["----------", "Rising Time 63%", "Rising Time 98%", "Failing Time 37%", "Output RMS", "Rcont"], index=w1671) -> (element=w1670:string)
                    n970 = call "fgv_status-display.vi"("Mode"=system-status."Update", "detail"=w1673, "title"=w1670) -> ()  [unwired: 8 in, 1 out]
                  }
                }
              }
            }
            frame #6 {
              # "size 14"
              # "size 7"
              # "size 7"
              # "디스플레이"
              n971 = Unbundle By Name(w1676) -> ("입력카운트"=w1686:dbl)
              n972 = Cluster To Array(cluster=w1676) -> (array=w1710:dbl[])
              n973 = global write "Global_params.vi" "measure_rc 동작"(w1676) -> ()
              n974 = To Long Integer(number=w1683) -> (32bit integer=w1681:i32)
              n975 = To Double Precision Float(number=w1712) -> (double precision float=w1709:dbl)
              n976 = Split 1D Array(array=w1710, index=2) -> (second subarray=w1708:dbl[])  [unwired: 1 out]
              n977 = Increment(x=w1709) -> ()  [unwired: 1 out]
              n978 = call "fgv_error_rc.vi"("cmd"=init-r-w."read") -> ("Error 2"=w1721:T16)  [unwired: 10 in]
              n979 = Unbundle By Name(w1721) -> ("제어단 단선"=w1720:bool, "제어단 단락"=w1719:bool, "제어단 특성변화"=w1718:bool, "출력단 단선"=w1717:bool, "출력단 단락"=w1716:bool, "출력단 특성변화"=w1715:bool, "온도"=w1714:bool)
              n980 = And Array Elements(Boolean array=w1691) -> (logical AND=w1690:bool)
              n981 = Select(t=w1686, s=w1690, f=0.0) -> (s? t:f=w1685:dbl)
              n982 = Build Array(w1686, w1685) -> (w1684:dbl[])
              n983 = Build Array(w1720, w1719, w1718, w1717, w1716, w1715, w1714) -> (w1707:bool[])
              n984 = call "count_run 1.vi"("cmd"=cmd_count."count", "CH"=w1681, "Array_Count"=w1684) -> ("Array_data"=w1682:dbl[][])  [unwired: 7 in, 1 out]
              n985 = Not(x=w1707) -> (.not. x?=w1724:bool[])
              n986 = Index Array(array=w1682, index (row)=w1681) -> (element=w1680:dbl[])  [unwired: 1 in]
              n987 = Index Array(array=w1680) -> (element #1=w1679:dbl, element #2=w1678:dbl)  [unwired: 2 in]
              n988 = Build Array (concatenate)(w1691, w1724) -> (w1693:bool[])
              n989 = Build Array (concatenate)(w1679, w1678, w1708) -> (w1677:dbl[])
              n990 = for {
                tunnel: w1693 -> [w1759] mode=indexing
                tunnel: [w1756] -> w1706 mode=indexing
                n991 = Select(t="OK", s=w1759, f="NG") -> (s? t:f=w1756:string)
              }
              n992 = Split 1D Array(array=w1677, index=14) -> (first subarray=w1722:dbl[])  [unwired: 1 out]
              n993 = And Array Elements(Boolean array=w1693) -> (logical AND=w1694:bool)
              n994 = for {
                tunnel: w1722 -> [w1730] mode=indexing
                tunnel: [w1729] -> w1697 mode=indexing
                tunnel: i16[] [0, 0, 0, 1, 1, 1, 1, 1, 1, 3, 1, 1, 1, 1] -> [w1728] mode=indexing
                n995 = Number To Fractional String(number=w1730, precision (6)=w1728) -> (F-format string=w1729:string)  [unwired: 2 in]
              }
              n996 = case shown="False" w1694 {
                tunnel: w1694 -> [w1746 _]
                tunnel: w1693 -> [w1745 _]
                frame False {
                  n997 = call "sub_shutdown.vi"("type"=shutdown-type."all") -> ()  [unwired: 10 in, 1 out]
                  n998 = for {
                    tunnel: w1746 -> [w1751]
                    tunnel: string[] ["제어단 단선", "제어단 단락", "제어단특성변화", "출력단 단선", "출력단 단락", "출력단 특성변화", "온도"] -> [w1750]
                    tunnel: w1745 -> [_] mode=indexing
                    i -> [w1749]
                    n999 = case shown="True" w1751 {
                      tunnel: w1750 -> [_ w1754]
                      tunnel: w1749 -> [_ w1753]
                      frame False {
                      }
                      frame True {
                        n1000 = Index Array(array=w1754, index=w1753) -> (element=w1752:string)
                        n1001 = call "sub_log_basic.vi"("desc"=w1752, "Title"="Shutdown ") -> ()  [unwired: 9 in, 1 out]
                      }
                    }
                  }
                }
                frame True {
                }
              }
              n1002 = Build Array (concatenate)(w1697, w1706) -> (w1695:string[])
              n1003 = call "fgv_error_rc.vi"("cmd"=init-r-w."read") -> ("Error 2"=w1704:T16)  [unwired: 10 in]
              n1004 = Unbundle By Name(w1704) -> ("제어단 단락"=w1701:bool, "출력단 단락"=w1700:bool)
              n1005 = Array Size(array=w1695) -> (size(s)=w1702:i32)
              n1006 = Initialize Array("-", w1702) -> (w1698:string[])
              n1007 = Or(x=w1701, y=w1700) -> (x .or. y?=w1699:bool)
              n1008 = Select(t=w1698, s=w1699, f=w1695) -> (s? t:f=w1696:string[])
              n1009 = case shown="True" w1699 {
                tunnel: [w1731 w1742] -> w1692
                tunnel: w1696 -> [w1731 w1744]
                tunnel: w1701 -> [_ w1740]
                tunnel: w1700 -> [_ w1732]
                frame False {
                }
                frame True {
                  n1010 = Select(t="NG", s=w1740, f="OK") -> (s? t:f=w1737:string)
                  n1011 = Replace Array Subset(array=w1744, new element=w1737, index=22) -> (w1743:string[])
                  n1012 = Select(t="NG", s=w1732, f="OK") -> (s? t:f=w1733:string)
                  n1013 = Replace Array Subset(array=w1743, new element=w1733, index=25) -> (w1742:string[])
                }
              }
              n1014 = call "TableCnt.vi"("cnt"=cmd_tablecnt."Write", "appended array"=w1692) -> ()  [unwired: 8 in, 2 out]
              n1015 = disable-structure shown="Disabled" {
                disable-tunnel: w1692 -> [w1726 _]
                frame Disabled {
                  n1016 = call "fgv_ngok_global.vi"("cmd"=rw."write", "results"=w1726) -> ()  [unwired: 9 in, 1 out]
                }
                frame Enabled {
                }
              }
            }
            frame #7 {
            }
          }
        }
      }
    }
  }
  "error out" <- "error in (no error)"
